vi "多道分析仪.vi"() -> ()   [LabVIEW 2014]
uses:
  <vilib>/Utility/miscctls.llb/LVPointDoubleTypeDef.ctl
  <vilib>/Utility/file.llb/Read From Spreadsheet File (DBL).vi
  <vilib>/Utility/file.llb/Write To Spreadsheet File (DBL).vi
  <vilib>/Analysis/NI_AAL_SigProc.lvlib
  <vilib>/Analysis/NI_AALPro.lvlib
panel:
  out "状态：本次测量和上次未完成测量时间和":dbl
  out "状态：本次测试已测时间":dbl
  out "状态：上次未完成测试的已测时间":dbl
  out "变量：每次测量计划用时":u16=3600
  out "设置：幅度谱总道数 2":u32=4096
  out "变量：实时计数":i32
  out "变量：剩余使用时间":dbl
  out "center":dbl caption="中心"
  in  "设置：信号极性（正T）":bool=TRUE
  in  "数据缓存索引":u32
  out "变量 : 实时总计数":u64
  out "设置 ： 修正文件路径":path
  out "变量 ： 上次测量总计数":u32
  out "变量：上次测量原始数据":dbl[](array[numeric])
  out "状态：已测时间":dbl
  out "状态：测量开始时间":u32
  out "状态：刷新次数":i32
  in  "状态：停止变量":bool=TRUE
  out "变量：上次测量时间":dbl
  out "变量：原始数据":dbl[](array[numeric])
  out "MCA道宽修正数组":ext[](array[numeric])
  in  "设置：寻峰灵敏度":i32=3 caption="宽度" min=3
  in  "设置：甄别前阈值":u16=10000
  in  "设置：甄别后阈值":u16=9000
  in  "设置：刷新频率":u16
  in  "设置：测量时间":u16
  out "结果：净面积":dbl=1313865.0
  out "结果：半高宽":dbl=218.0
  out "结果：峰位":dbl=1585.0 caption="中心"
  in  "按钮_游标":bool caption="游标"
  in  "按钮_寻峰":T1 caption="寻峰"
  in  "按钮_右移":bool caption="右移"
  in  "按钮_还原":bool caption="还原"
  in  "按钮_放大":bool caption="放大"
  in  "按钮_左移":bool caption="左移"
  out "变量：感兴区终点道址":dbl=-1.0
  in  "显示：列表显示内容":string[](array[string])=["", "0秒", "正", "9000", "10000", "", "", "2014年3月7日", "0:56:44", "0秒", "0", "", "", "", "", "", "", "", "", "", "", ""]
  out "变量：感兴区起点道址":dbl=-1.0
  out "设置：幅度谱总道数":u32=4096
  in  "变量：图像缓存数组":dbl[][](array[numeric])
  in  "按钮_退出":bool caption="退出"
  in  "按钮_帮助":bool caption="帮助"
  in  "按钮_复位":bool caption="复位"
  in  "按钮_停止":bool caption="停止"
  in  "按钮_开始":bool caption="开始"
  in  "按钮_设置":bool caption="设置"
  in  "按钮_保存":bool caption="保存"
  in  "按钮_打开":bool caption="打开"
  out "显示：波形图":dbl[][](graph)
  out "显示：列表框":T2=6
  out "显示：波形图_预览":dbl[][](graph)
  out "状态栏_仪器状态":T3="核电子学硬件平台未连接" caption="状态栏"
  out "状态栏_剩余使用时间":T3="0" caption="剩余使用时间："
  out "状态栏_计数率":T3="0" caption="实时计数率："
  out "状态栏_游标状态":T3="隐藏" caption="游标状态："
  out "状态栏_游标计数":T3="0" caption="游标计数："
  out "状态栏_游标道址":T3="0" caption="游标道址："
  out "状态栏_测量状态":T3="停止" caption="测量状态："
  out "状态栏_日期":T3="2014/3/7   0:56:56" caption="日期"
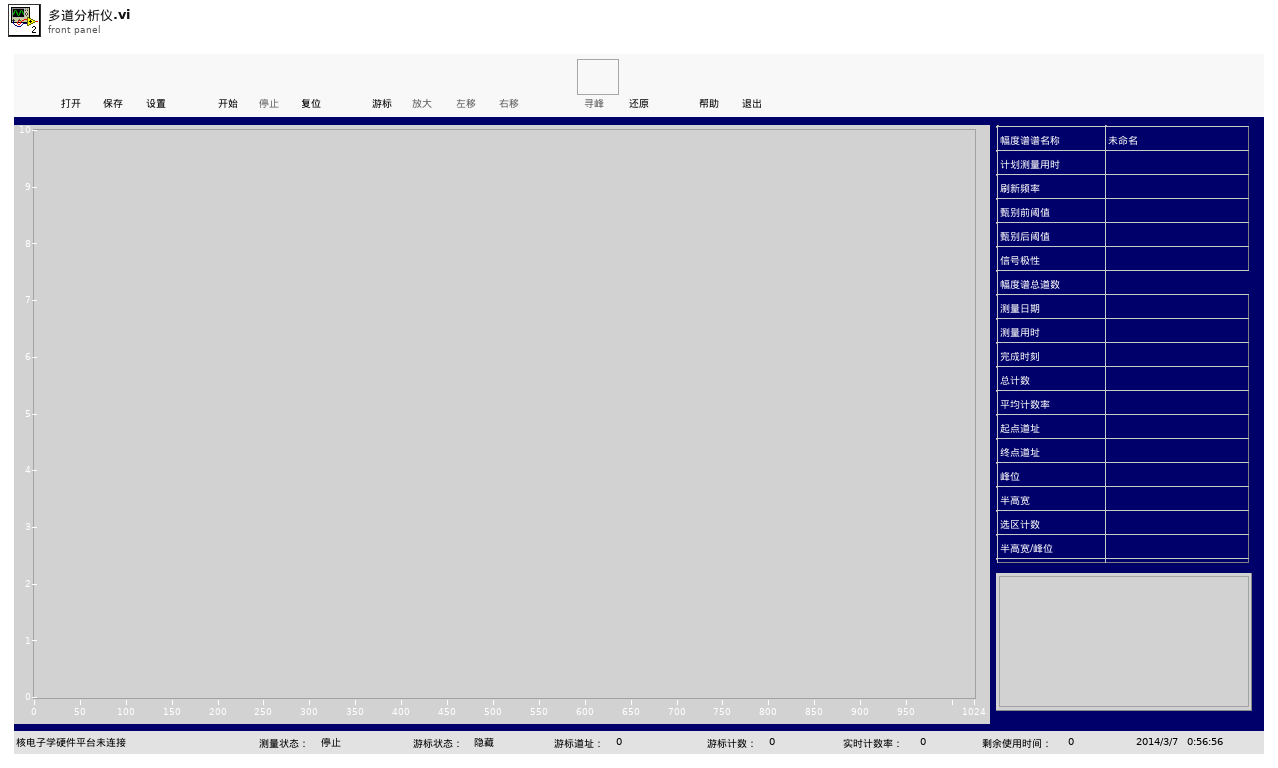
[diagram p1: front panel]
types:
  T1 = typedef "寻峰控件.ctl" = bool
  T2 = typedef "透明表格.ctl" = i32
  T3 = typedef "透明字符串.ctl" = string
  T4 = typedef "枚举常量_状态机.ctl" = enum16{"初始化", "等待", "完成"}
  T5 = typedef "LVPointDoubleTypeDef.ctl" = cluster{"X":dbl, "Y":dbl}
  T6 = enum8{"Enabled", "Disabled", "Disabled and Grayed Out"}
  T7 = enum16{"open", "open or create", "create or replace", "create", "open (read-only)"}
  T8 = typedef "eventvkey.ctl" = enum16{"ASCII", "Enter", "Return", "Shift", "Ctrl", "Alt", "Cmd", "Opt", "Caps", "NumLock", "Clear", "Break", "Up", "Down", "Left", "Right", "Insert", "Delete", "Home", "End", "PageUp", "PageDown", "Escape", "Help", "Pause", "ScrollLock", "F1", "F2", "F3", "F4", "F5", "F6", "F7", "F8", "F9", "F10", "F11", "F12", "F13", "F14", "F15", "F16", "F17", "F18", "F19", "F20", "F21", "F22", "F23", "F24", "Play", "VolumeUp", "VolumeDown", "Mute", "Two Byte Char"}
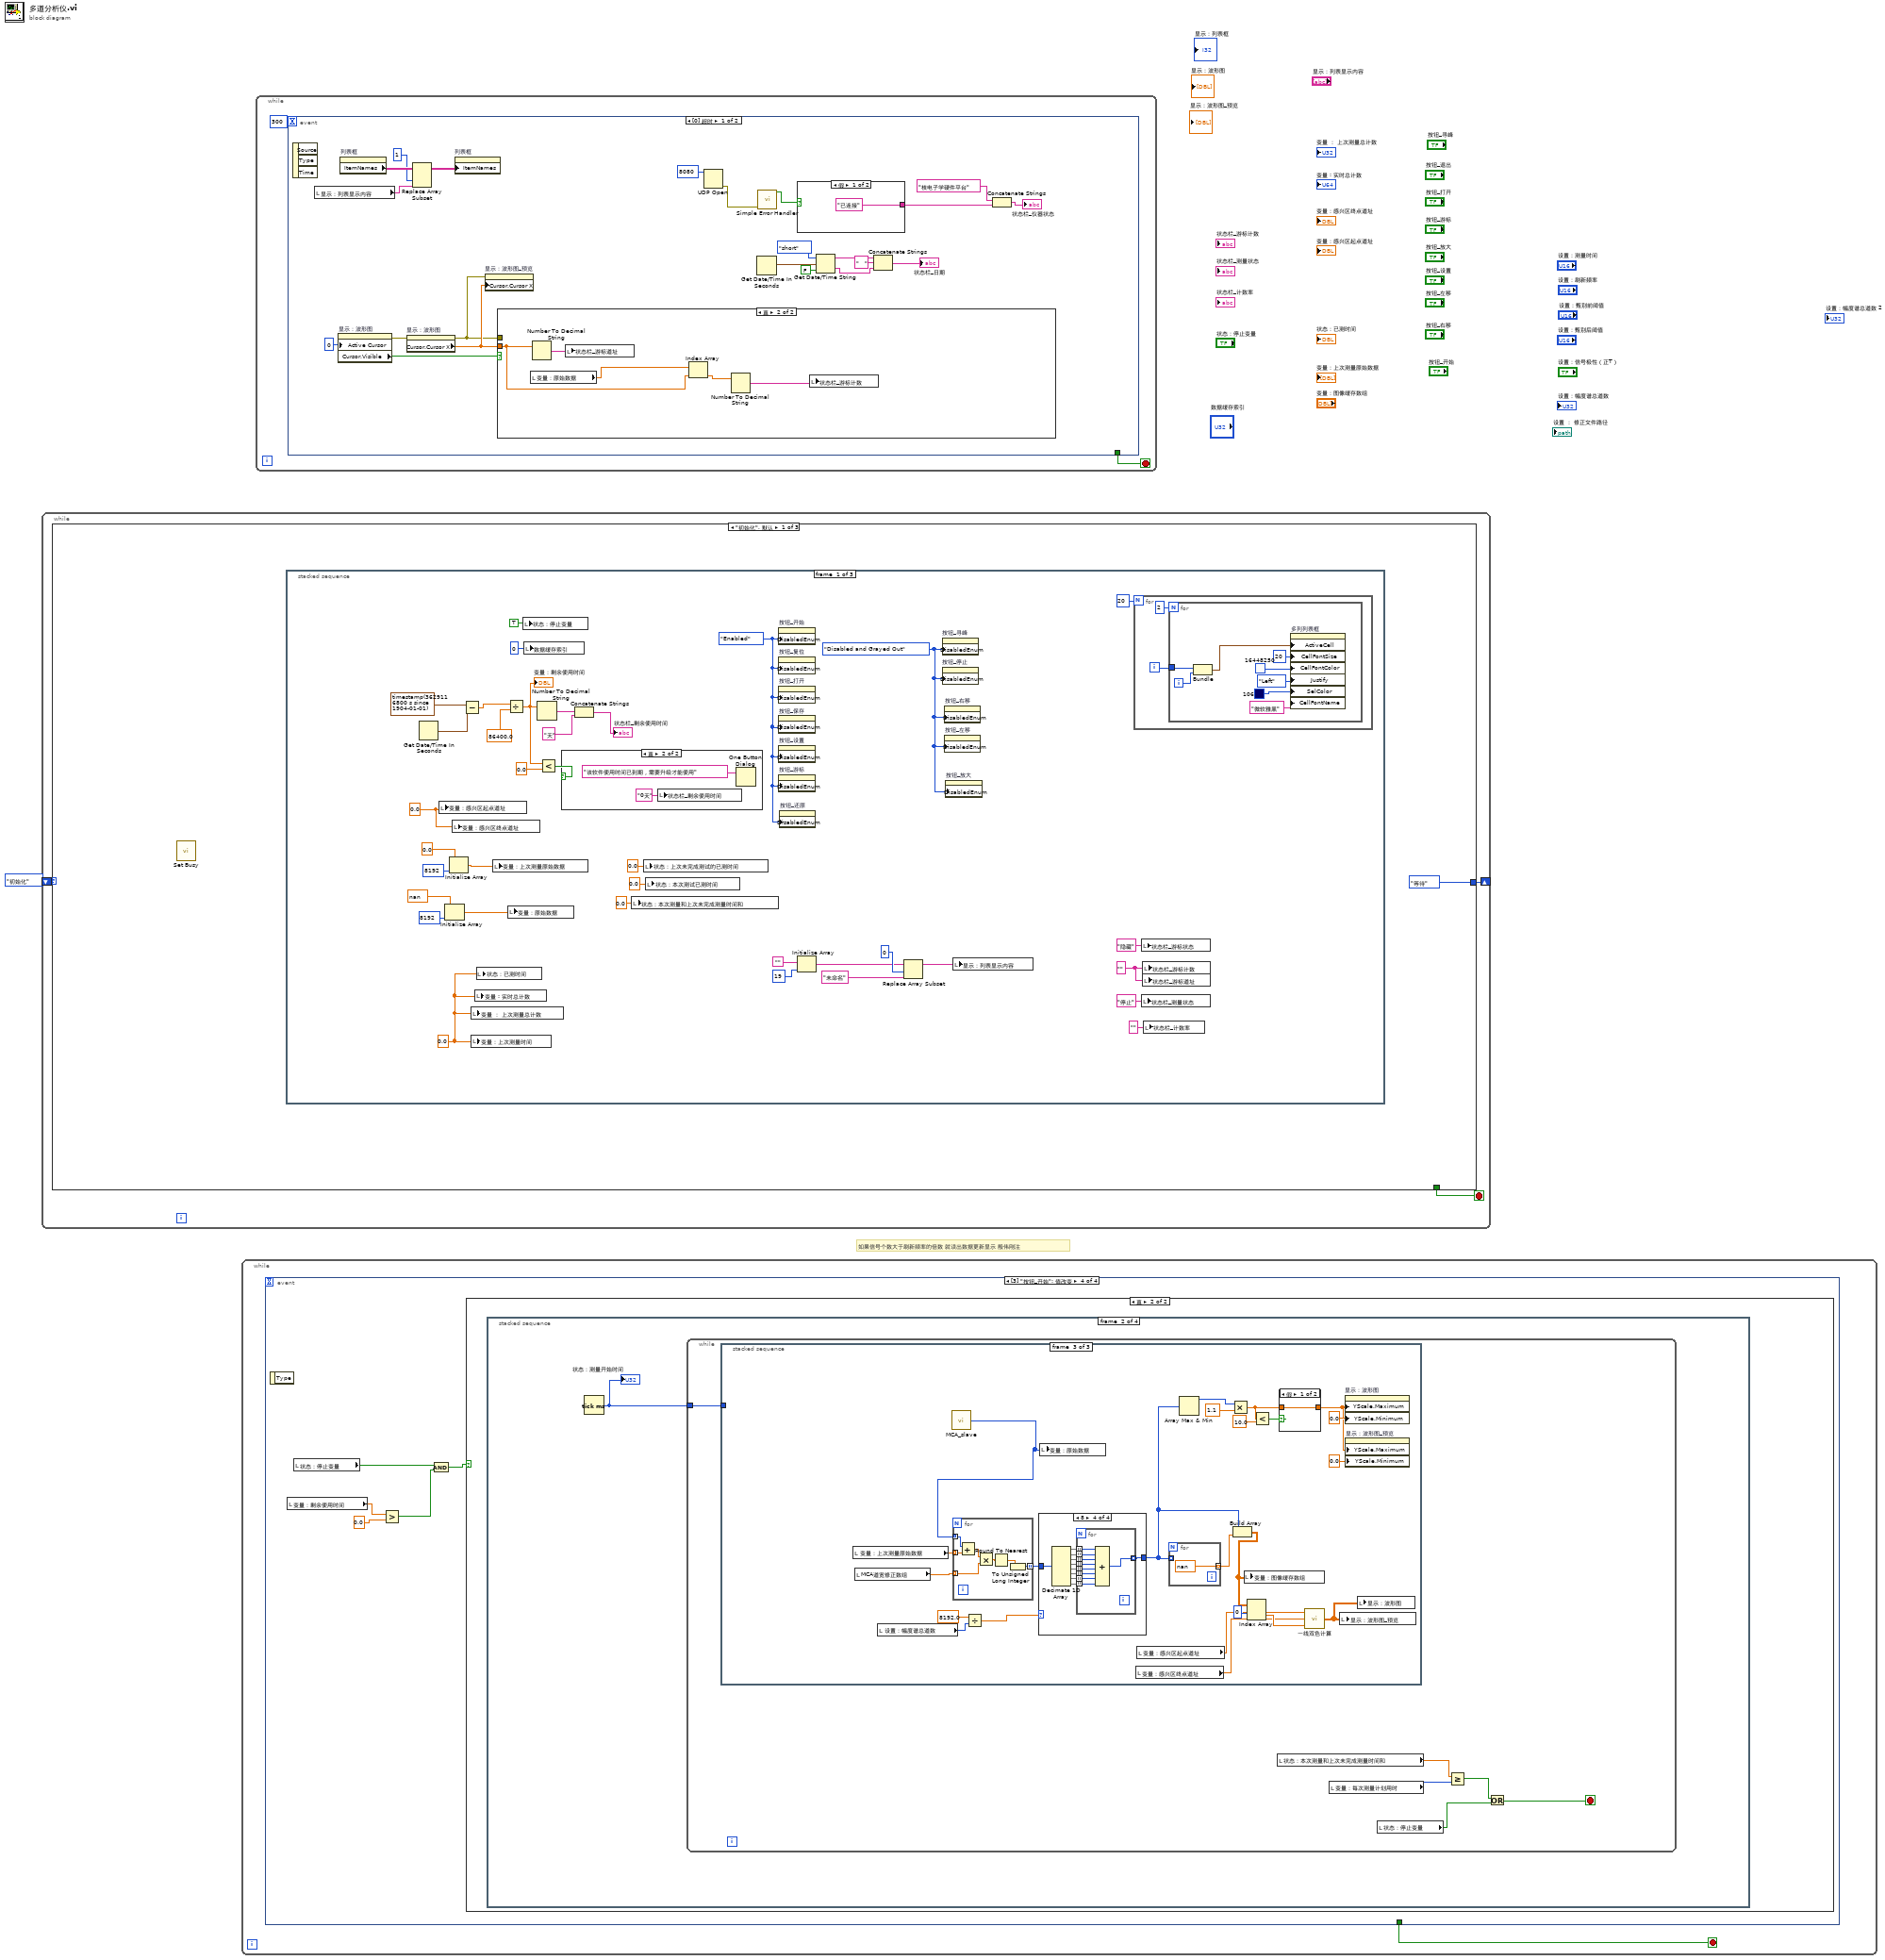
[diagram p0: block diagram]
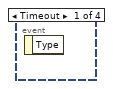
[diagram p2: hidden frame]
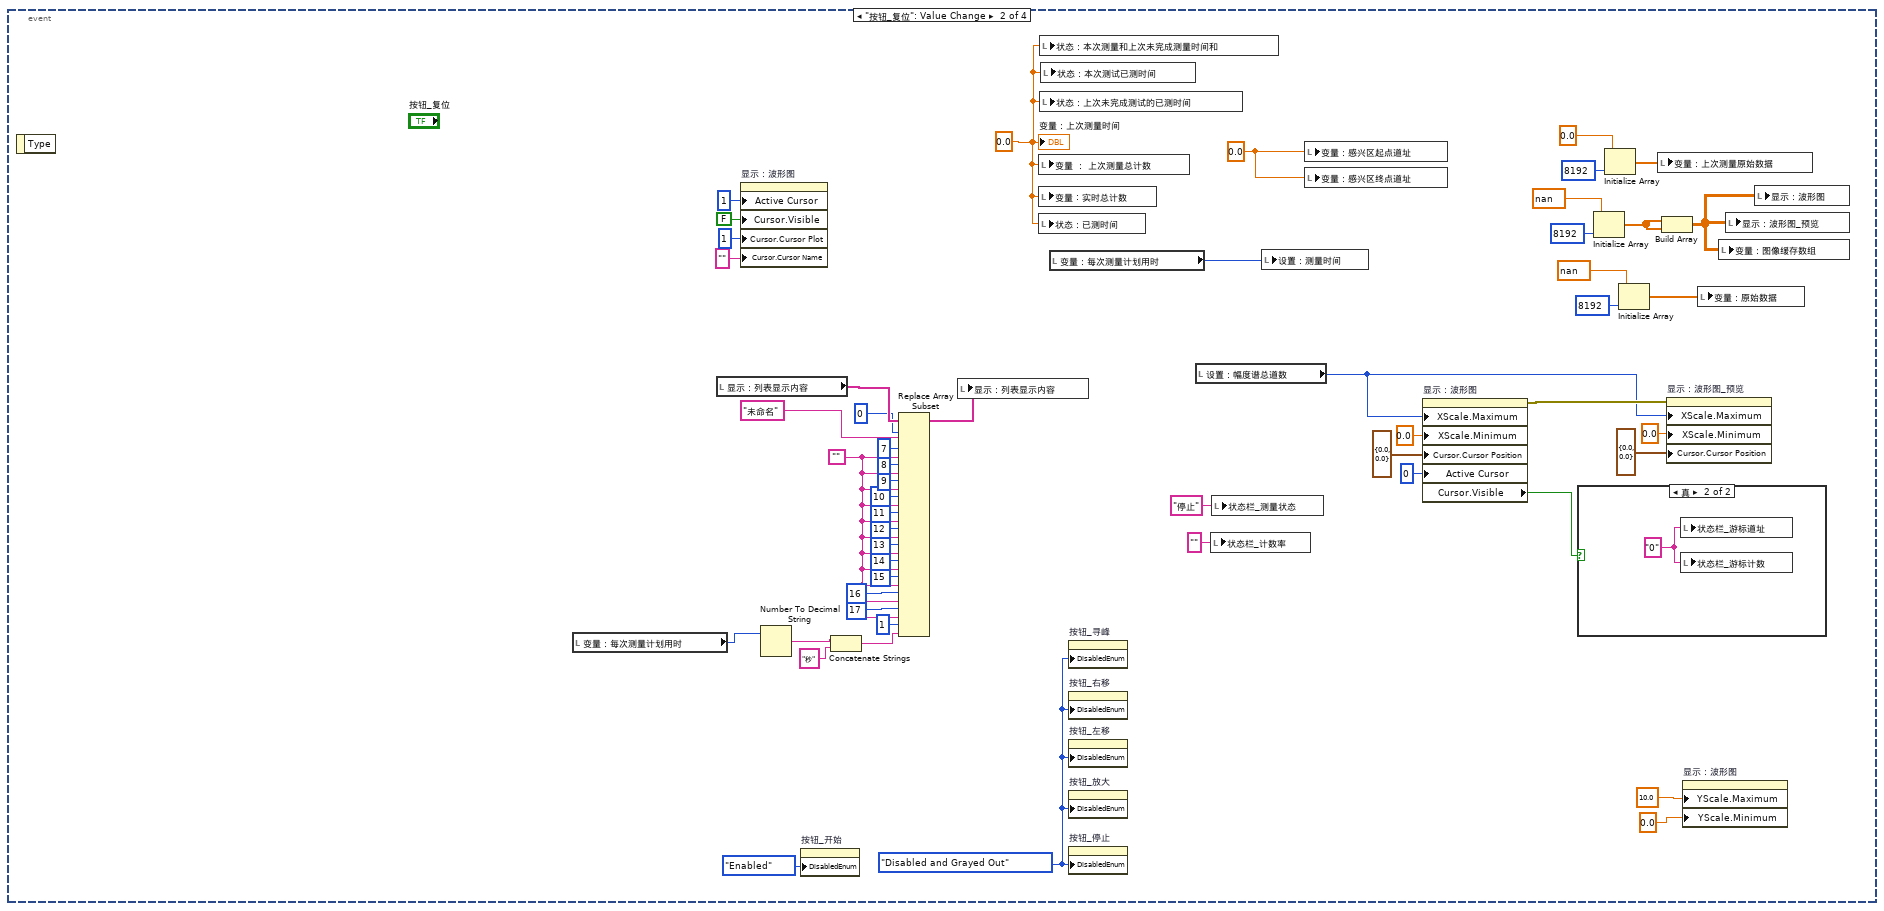
[diagram p3: hidden frame]
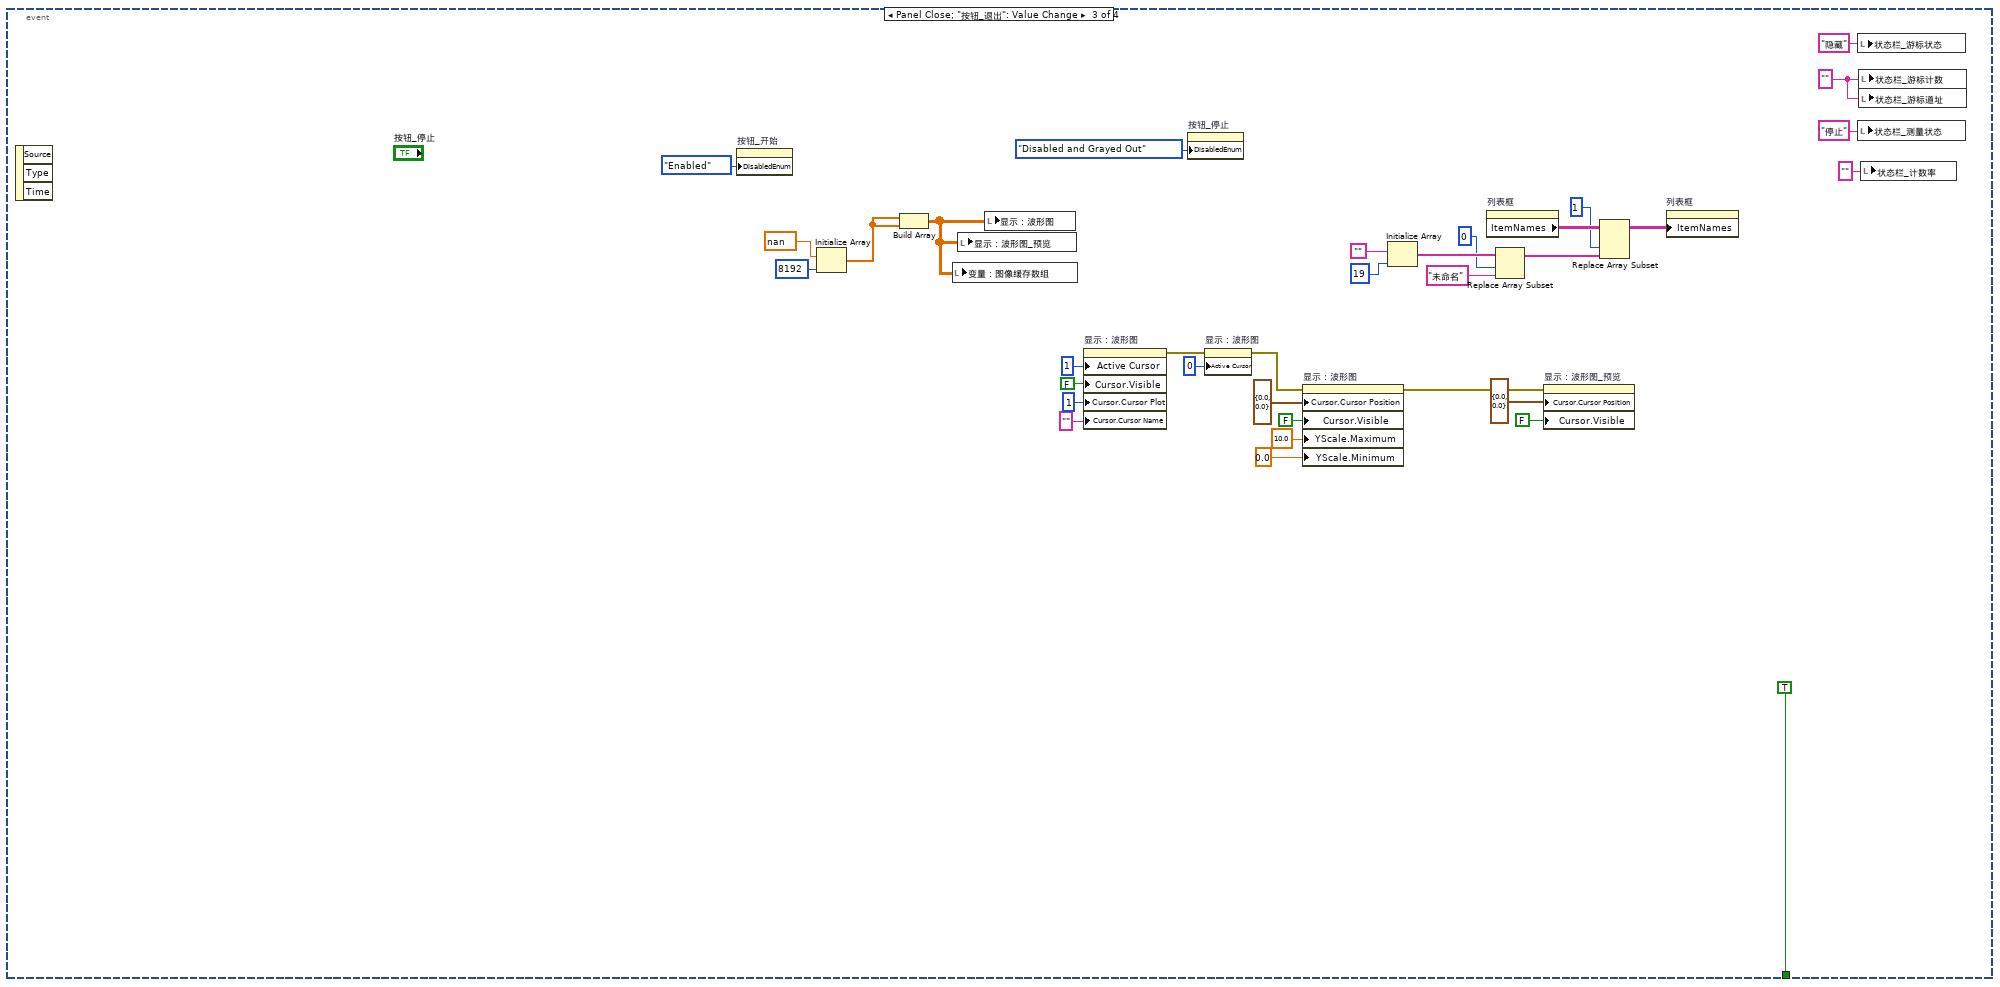
[diagram p5: hidden frame]
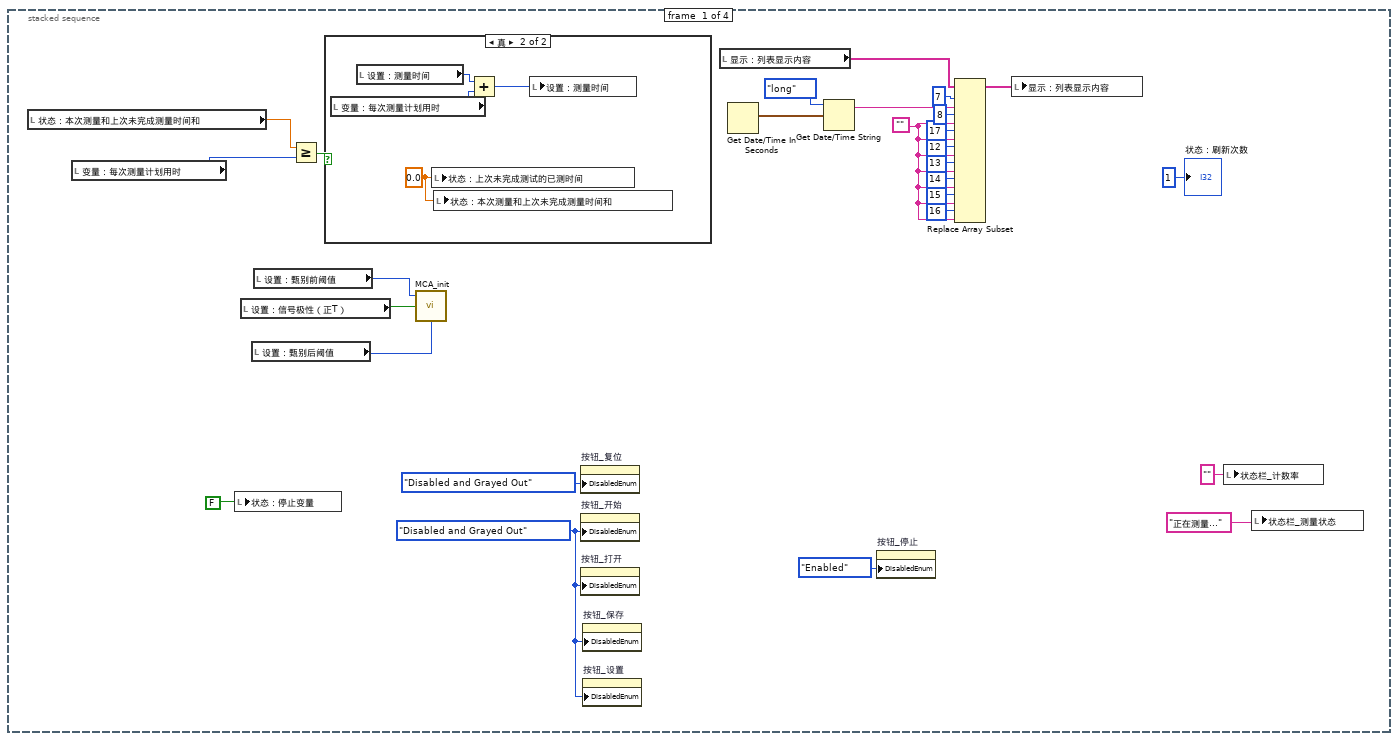
[diagram p7: hidden frame]
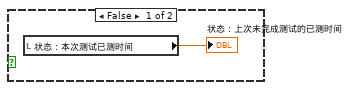
[diagram p8: hidden frame]
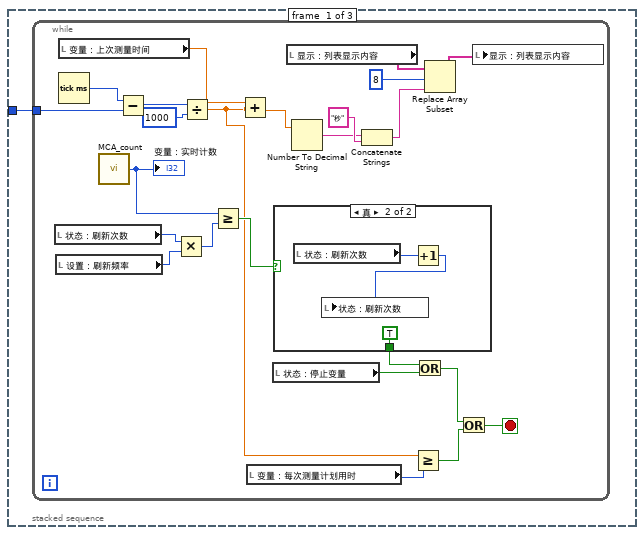
[diagram p9: hidden frame]
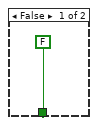
[diagram p10: hidden frame]
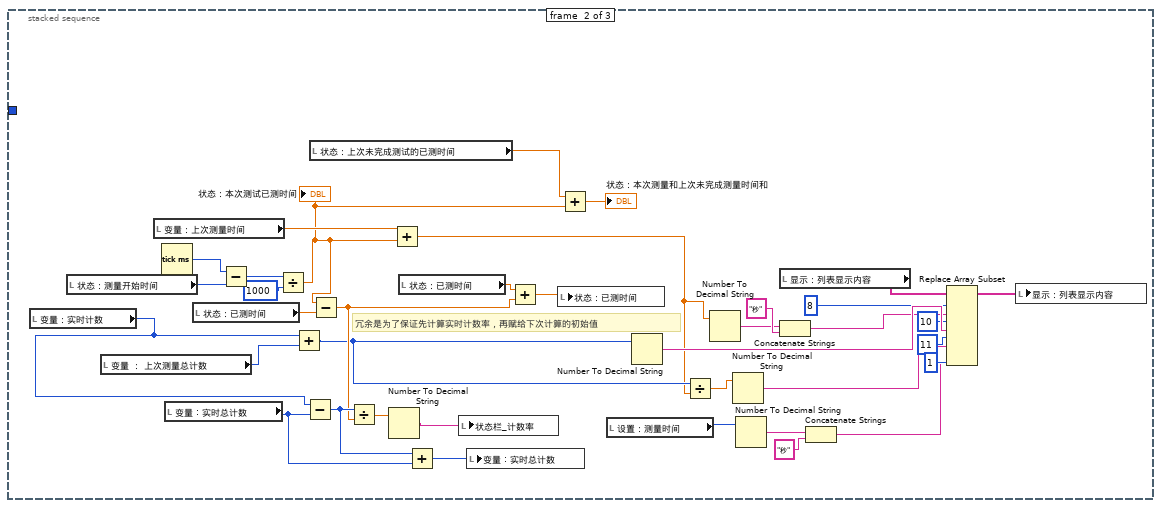
[diagram p11: hidden frame]
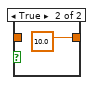
[diagram p12: hidden frame]
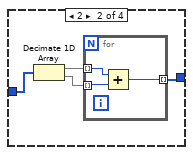
[diagram p14: hidden frame]
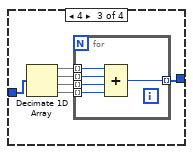
[diagram p15: hidden frame]
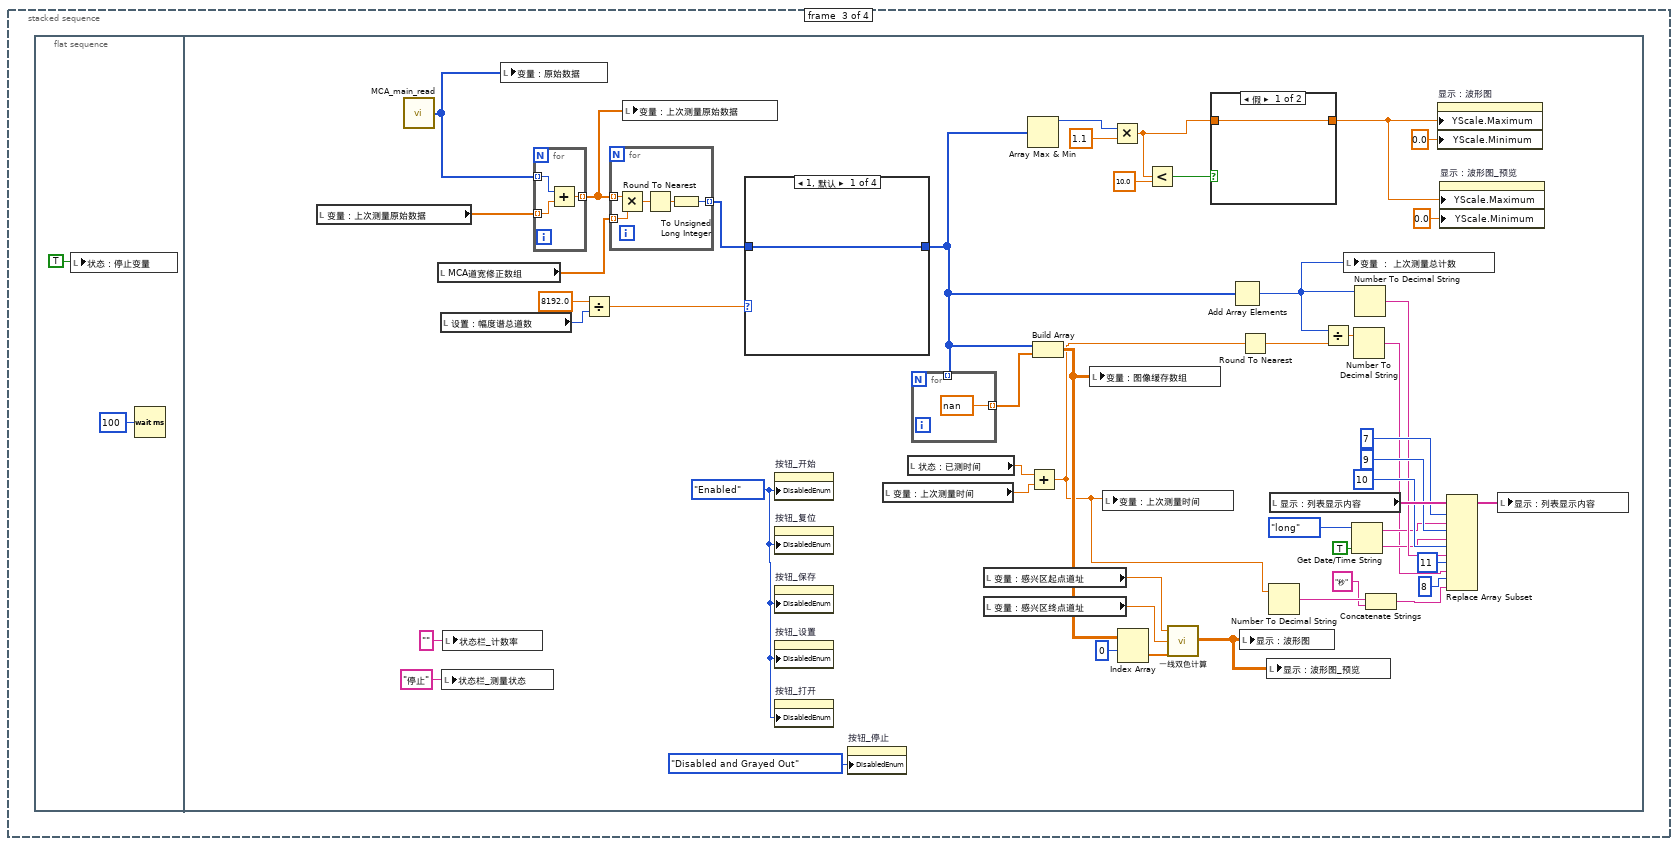
[diagram p16: hidden frame]
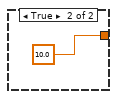
[diagram p17: hidden frame]
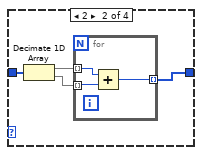
[diagram p18: hidden frame]
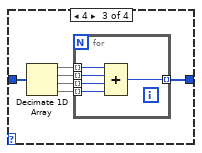
[diagram p19: hidden frame]
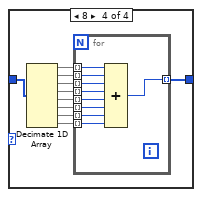
[diagram p20: hidden frame]
diagram:
  # "如果信号个数大于刷新频率的倍数 就读出数据更新显示 殷伟刚注"
  n1 = while {
    shift-right: [w3] -> _
    shift-left: 枚举常量_状态机."初始化" ("枚举") -> [w4]
    stop <- w2 stop-if-true
    n2 = case shown="\"初始化\", 默认" w4 {
      tunnel: [枚举常量_状态机."等待" ("枚举") w121 枚举常量_状态机."完成" ("枚举")] -> w3
      tunnel: [_ _ TRUE] -> w2
      frame "初始化", Default {
        n3 = call <vilib>:"Set Busy.vi"() -> ()  [unwired: 10 in, 2 out]
        n4 = stacked-sequence {
          frame #0 {
            w28 = 0.0
            w25 = 0.0 ("变量：已测量时间")
            w30 = T6."Enabled" ("禁用")
            w38 = T3 "" ("状态栏_游标计数")
            w20 = T6."Disabled and Grayed Out" ("禁用")
            n5 = Get Date/Time In Seconds() -> (seconds since 1Jan1904=w12:timestamp)
            n6 = local write "变量：感兴区起点道址"(w28) -> ()
            n7 = Initialize Array(nan ("元素"), 8192 ("维数大小")) -> (w21:dbl[])
            n8 = Initialize Array(0.0 ("元素"), 8192 ("维数大小")) -> (w24:dbl[])
            n9 = local write "变量：感兴区终点道址"(w28) -> ()
            n10 = Subtract(x=timestamp(3629116800 s since 1904-01-01), y=w12) -> (x-y=w14:dbl)
            n11 = local write "变量 ： 上次测量总计数"(w25) -> ()
            n12 = local write "变量：上次测量时间"(w25) -> ()
            n13 = local write "变量 : 实时总计数"(w25) -> ()
            n14 = local write "状态：已测时间"(w25) -> ()
            n15 = local write "变量：上次测量原始数据"(w24) -> ()
            n16 = Divide(x=w14, y=86400.0) -> (x/y=w11:dbl)
            "变量：剩余使用时间" <- w11
            n17 = local write "变量：原始数据"(w21) -> ()
            n18 = local write "状态：停止变量"(TRUE ("停止变量")) -> ()
            n19 = local write "数据缓存索引"(u32 0 ("数据缓存索引")) -> ()
            n20 = Number To Decimal String(number=w11) -> (decimal integer string=w16:string)  [unwired: 1 in]
            n21 = Less?(x=w11, y=0.0) -> (x < y?=w9:bool)
            n22 = case shown="真" w9 {
              frame False {
              }
              frame True {
                n23 = local write "状态栏_剩余使用时间"(T3 "0天" ("状态栏_剩余使用时间")) -> ()
                n24 = One Button Dialog(message="该软件使用时间已到期，需要升级才能使用" ("消息")) -> ()  [unwired: 1 in, 1 out]
              }
            }
            n25 = Concatenate Strings(w16, "天" ("字符串")) -> (→"状态栏_剩余使用时间":string)
            n26 = local write "状态：本次测量和上次未完成测量时间和"(0.0 ("状态：本次测量和上次未完成测量时间和")) -> ()
            n27 = local write "状态：上次未完成测试的已测时间"(0.0 ("状态：上次未完成测试的已测时间")) -> ()
            n28 = local write "状态：本次测试已测时间"(0.0 ("状态：本次测试已测时间")) -> ()
            n29 = property on="按钮_开始" class="Bool"("DisabledEnum"=w30) -> ()  [unwired: 2 in, 2 out]
            n30 = property on="按钮_复位" class="Bool"("DisabledEnum"=w30) -> ()  [unwired: 2 in, 2 out]
            n31 = property on="按钮_打开" class="Bool"("DisabledEnum"=w30) -> ()  [unwired: 2 in, 2 out]
            n32 = property on="按钮_保存" class="Bool"("DisabledEnum"=w30) -> ()  [unwired: 2 in, 2 out]
            n33 = property on="按钮_设置" class="Bool"("DisabledEnum"=w30) -> ()  [unwired: 2 in, 2 out]
            n34 = property on="按钮_游标" class="Bool"("DisabledEnum"=w30) -> ()  [unwired: 2 in, 2 out]
            n35 = property on="按钮_还原" class="Bool"("DisabledEnum"=w30) -> ()  [unwired: 2 in, 2 out]
            n36 = Initialize Array("", 19 ("维数大小")) -> (w31:string[])
            n37 = Replace Array Subset(array=w31, new element="未命名" ("新元素/子数组"), index=0 ("索引")) -> (w36:string[])
            n38 = property on="按钮_寻峰" class="Bool"("DisabledEnum"=w20) -> ()  [unwired: 2 in, 2 out]
            n39 = property on="按钮_停止" class="Bool (严格)"("DisabledEnum"=w20) -> ()  [unwired: 2 in, 2 out]
            n40 = property on="按钮_右移" class="Bool"("DisabledEnum"=w20) -> ()  [unwired: 2 in, 2 out]
            n41 = property on="按钮_左移" class="Bool"("DisabledEnum"=w20) -> ()  [unwired: 2 in, 2 out]
            n42 = property on="按钮_放大" class="Bool"("DisabledEnum"=w20) -> ()  [unwired: 2 in, 2 out]
            n43 = local write "显示：列表显示内容"(w36) -> ()
            n44 = for {
              N: 20 -> [_]
              i -> [w44]
              n45 = for {
                N: 2 -> [_]
                tunnel: w44 -> [w52]
                i -> [w53]
                n46 = Bundle(w52, w53) -> (w51:cluster{i32, i32})  [unwired: 1 in]
                n47 = property on="多列列表框" class="MCListbox (严格)"("ActiveCell"=w51, "CellFontSize"=u32 20 ("活动单元格:单元格字体:字号"), "CellFontColor"=u32 16448250 ("Color"), "Justify"=enum16{"Left", "Center", "Right"}."Left" ("活动单元格:单元格对齐"), "SelColor"=u32 106 ("Color"), "CellFontName"="微软雅黑" ("活动单元格:单元格字体:名称")) -> ()  [unwired: 2 in, 2 out]
              }
            }
            n48 = local write "状态栏_游标状态"(T3 "隐藏" ("状态栏_游标状态")) -> ()
            n49 = local write "状态栏_测量状态"(T3 "停止" ("状态栏_测量状态")) -> ()
            n50 = local write "状态栏_游标计数"(w38) -> ()
            n51 = local write "状态栏_游标道址"(w38) -> ()
            n52 = local write "状态栏_计数率"(T3 "" ("状态栏_计数率")) -> ()
          }
          frame #1 {
            # "此处得到MCA道宽不均匀修正数组"
            n53 = call "MCA_ReadConfig.vi"() -> ("数据刷新频率"=w57:u16, "测量最多花费的时间（秒）："=w58:u16, "甄别后阈值"=w59:u16, "甄别前阈值"=w60:u16, "寻峰灵敏度"=w56:u16, "最大道数"=w54:u16, "数据文件路径"=w55:path, "信号极性"=w61:bool)  [unwired: 3 in, 1 out]
            "变量：每次测量计划用时" <- w58
            n54 = local write "设置：信号极性（正T）"(w61) -> ()
            n55 = local write "设置：幅度谱总道数"(w54) -> ()
            n56 = local write "设置：甄别前阈值"(w60) -> ()
            n57 = local write "设置：甄别后阈值"(w59) -> ()
            n58 = local write "设置：测量时间"(w58) -> ()
            n59 = local write "设置：刷新频率"(w57) -> ()
            n60 = local write "设置：寻峰灵敏度"(w56) -> ()
            n61 = Equal?(x=w55, y=path "") -> (x = y?=w83:bool)
            n62 = case shown="真" w83 {
              tunnel: w55 -> [w88 _]
              tunnel: [w86 w89] -> w62
              frame False {
                n63 = call-poly <vilib>:"Read From Spreadsheet File.vi"("transpose (no:F)"=TRUE, "file path (dialog if empty)"=w88) -> ("first row"=w86:dbl[])  [unwired: 5 in, 4 out]
              }
              frame True {
                n64 = Initialize Array(1.0 ("元素"), 8192 ("维数大小")) -> (w89:dbl[])
              }
            }
            "MCA道宽修正数组" <- w62
            n65 = local write "设置 ： 修正文件路径"(w55) -> ()
            n66 = property on="显示：波形图" class="WFGraph (严格)"("Active Cursor"=u32 1 ("活动游标"), "Cursor.Visible"=FALSE ("游标.可见"), "Cursor.Cursor Plot"=1 ("游标.游标关联曲线"), "Cursor.Cursor Name"="" ("游标.游标名")) -> (error out=w66:errorcluster)  [unwired: 2 in, 1 out]
            n67 = property on="显示：波形图" class="WFGraph (严格)"(error in=w66, "Active Cursor"=u32 0 ("活动游标")) -> (error out=w71:errorcluster)  [unwired: 1 in, 1 out]
            n68 = property on="显示：波形图" class="WFGraph (严格)"(error in=w71, "XScale.Maximum"=w54, "XScale.Minimum"=0.0 ("X标尺.范围:最小值"), "Cursor.Cursor Position"=T5 {"X"=0.0, "Y"=0.0} ("游标.游标位置"), "Cursor.Visible"=FALSE ("游标.可见"), "YScale.Maximum"=10.0 ("Y标尺.范围:最大值"), "YScale.Minimum"=0.0 ("Y标尺.范围:最小值")) -> (error out=w74:errorcluster)  [unwired: 1 in, 1 out]
            n69 = Initialize Array(nan ("元素"), w54) -> (w82:dbl[])
            n70 = for {
              tunnel: w82 -> [_] mode=indexing
              tunnel: [nan] -> w79 mode=indexing
            }
            n71 = property on="显示：波形图_预览" class="WFGraph (严格)"(error in=w74, "XScale.Maximum"=w54, "XScale.Minimum"=0.0 ("X标尺.范围:最小值"), "Cursor.Cursor Position"=T5 {"X"=0.0, "Y"=0.0} ("游标.游标位置"), "Cursor.Visible"=FALSE ("游标.可见")) -> ()  [unwired: 1 in, 2 out]
            n72 = Build Array(w82, w79) -> (w80:dbl[][])
            n73 = local write "显示：波形图_预览"(w80) -> ()
            n74 = local write "变量：图像缓存数组"(w80) -> ()
            n75 = local write "显示：波形图"(w80) -> ()
          }
          frame #2 {
            n76 = local read "设置：信号极性（正T）"() -> (w99:bool)
            n77 = local read "设置：寻峰灵敏度"() -> (w102:i32)
            n78 = local read "设置：幅度谱总道数"() -> (w94:u32)
            n79 = local read "设置：测量时间"() -> (w106:u16)
            n80 = local read "设置：刷新频率"() -> (w105:u16)
            n81 = local read "设置：甄别后阈值"() -> (w103:u16)
            n82 = local read "设置：甄别前阈值"() -> (w104:u16)
            n83 = case shown="假" w99 {
              tunnel: ["负" ("字符串") "正" ("字符串")] -> w98
              frame False {
              }
              frame True {
              }
            }
            n84 = Number To Decimal String(number=w102) -> (decimal integer string=w96:string)  [unwired: 1 in]
            n85 = Number To Decimal String(number=w94) -> (decimal integer string=w93:string)  [unwired: 1 in]
            n86 = Number To Decimal String(number=w106) -> (decimal integer string=w111:string)  [unwired: 1 in]
            n87 = Number To Decimal String(number=w103) -> (decimal integer string=w100:string)  [unwired: 1 in]
            n88 = Number To Decimal String(number=w105) -> (decimal integer string=w116:string)  [unwired: 1 in]
            n89 = Number To Decimal String(number=w104) -> (decimal integer string=w101:string)  [unwired: 1 in]
            n90 = Concatenate Strings(w111, "秒" ("字符串")) -> (w112:string)
            n91 = Concatenate Strings(w116, "个/次" ("字符串")) -> (w118:string)
            n92 = local read "显示：列表显示内容"() -> (w108:string[])
            n93 = Replace Array Subset(array=w108, new element #1=w112, index #1=1 ("索引"), new element #2=w118, index #2=2 ("索引"), new element #3=w101, index #3=3 ("索引"), new element #4=w100, index #4=4 ("索引"), new element #5=w98, index #5=5 ("索引"), new element #6=w93, index #6=6 ("索引"), new element #7=w96, index #7=18 ("索引")) -> (w109:string[])
            n94 = local write "显示：列表显示内容"(w109) -> ()
          }
        }
      }
      frame "等待" {
        n95 = call <vilib>:"Unset Busy.vi"() -> ()  [unwired: 11 in, 1 out]
        n96 = event shown="[5] \"按钮_打开\": 值改变" {
          selector: _ -> [_ _ _ _ _ _ _ _ _ _ _ _ _ _ _ _ _]
          dyn-events: _ -> [_ _ _ _ _ _ _ _ _ _ _ _ _ _ _ _ _]
          timeout: _ -> [_ _ _ _ _ _ _ _ _ _ _ _ _ _ _ _ _]
          tunnel: [枚举常量_状态机."等待" ("枚举") 枚举常量_状态机."等待" ("枚举") 枚举常量_状态机."完成" ("枚举") 枚举常量_状态机."等待" ("枚举") 枚举常量_状态机."等待" ("枚举") 枚举常量_状态机."等待" ("枚举") 枚举常量_状态机."等待" ("枚举") 枚举常量_状态机."等待" ("枚举") 枚举常量_状态机."等待" ("枚举") 枚举常量_状态机."等待" ("枚举") 枚举常量_状态机."等待" ("枚举") 枚举常量_状态机."等待" ("枚举") 枚举常量_状态机."等待" ("枚举") 枚举常量_状态机."等待" ("枚举") 枚举常量_状态机."等待" ("枚举") 枚举常量_状态机."等待" ("枚举") 枚举常量_状态机."等待" ("枚举")] -> w121
          event Timeout {
            n97 = event-data() -> ()  [unwired: 1 in, 3 out]
          }
          event "按钮_帮助": Value Change {
            n98 = event-data() -> ()  [unwired: 1 in, 6 out]
            n99 = call "显示对话框信息"() -> ("软件介绍"=w123:bool)  [unwired: 10 in, 1 out]
            n100 = case shown="真" w123 {
              frame False {
              }
              frame True {
                n101 = call "显示对话框信息2"() -> ()  [unwired: 10 in, 2 out]
              }
            }
          }
          event "按钮_退出": Value Change {
            n102 = event-data() -> ()  [unwired: 1 in, 6 out]
            n103 = local write "状态：停止变量"(TRUE ("停止变量")) -> ()
          }
          event "按钮_停止": Value Change {
            w130 = T6."Enabled" ("禁用")
            n104 = event-data() -> ()  [unwired: 1 in, 6 out]
            n105 = property on="按钮_复位" class="Bool"("DisabledEnum"=w130) -> ()  [unwired: 2 in, 2 out]
            n106 = property on="按钮_开始" class="Bool"("DisabledEnum"=T6."Enabled" ("禁用")) -> ()  [unwired: 2 in, 2 out]
            n107 = property on="按钮_打开" class="Bool"("DisabledEnum"=w130) -> ()  [unwired: 2 in, 2 out]
            n108 = property on="按钮_保存" class="Bool"("DisabledEnum"=w130) -> ()  [unwired: 2 in, 2 out]
            n109 = property on="按钮_设置" class="Bool"("DisabledEnum"=w130) -> ()  [unwired: 2 in, 2 out]
            n110 = local write "状态：停止变量"(TRUE ("停止变量")) -> ()
            n111 = property on="按钮_停止" class="Bool (严格)"("Value"=FALSE ("停止"), "DisabledEnum"=T6."Disabled and Grayed Out" ("禁用")) -> ()  [unwired: 2 in, 2 out]
          }
          event "显示：波形图": Cursor Move {
            n112 = event-data() -> ()  [unwired: 1 in, 9 out]
            n113 = property on="显示：波形图" class="WFGraph (严格)"() -> ("Cursor.Cursor Position"=w140:T5)  [unwired: 2 in, 2 out]
            n114 = property on="显示：波形图_预览" class="WFGraph (严格)"("Cursor.Cursor Position"=w140) -> ()  [unwired: 2 in, 2 out]
            n115 = Unbundle By Name(w140) -> ("Cursor X"=w137:dbl, "Cursor Y"=w136:dbl)
            n116 = Number To Decimal String(number=w137) -> (decimal integer string=→"状态栏_游标道址":string)  [unwired: 1 in]
            n117 = Number To Decimal String(number=w136) -> (decimal integer string=w135:string)  [unwired: 1 in]
            n118 = Equal?(x=w135, y="NaN") -> (x = y?=w141:bool)
            n119 = case shown="真" w141 {
              tunnel: [w143 w149] -> w138
              tunnel: w136 -> [w143 _]
              frame False {
              }
              frame True {
                n120 = property on="显示：波形图" class="WFGraph (严格)"() -> (error out=w150:errorcluster, "Cursor.Cursor Plot"=w146:i32)  [unwired: 2 in, 1 out]
                n121 = Equal To 0?(x=w146) -> (x = 0?=w147:bool)
                n122 = Select(t=1.0, s=w147, f=0.0) -> (s? t:f=w148:dbl)
                n123 = property on="显示：波形图" class="WFGraph (严格)"(error in=w150, "Cursor.Cursor Plot"=w148) -> ("Cursor.Cursor Y"=w149:dbl)  [unwired: 1 in, 2 out]
              }
            }
            n124 = Number To Decimal String(number=w138) -> (decimal integer string=w133:string)  [unwired: 1 in]
            n125 = local write "状态栏_游标计数"(w133) -> ()
          }
          event "按钮_打开": Value Change {
            n126 = event-data() -> ()  [unwired: 1 in, 1 out]
            n127 = call "MCA_OpenDialog.vi"() -> ("要打开的数据文件路径： 2"=w151:path, "是否取消？"=w152:bool)  [unwired: 10 in]
            n128 = case shown="假" w152 {
              tunnel: w151 -> [w154 _]
              frame False {
                n129 = Strip Path(path=w154) -> (name=w161:string)  [unwired: 1 out]
                n130 = String Length(string=w161) -> (length=w160:i32)
                n131 = Subtract(x=w160, y=4) -> (x-y=w158:i32)
                n132 = String Subset(string=w161, offset (0)=w158, length (rest)=w160) -> (substring=w157:string)
                n133 = Equal?(x=w157, y="tdms") -> (x = y?=w155:bool)
                n134 = case shown="真" w155 {
                  tunnel: w154 -> [w163 w195]
                  frame False {
                    n135 = Strip Path(path=w163) -> (name=w162:string)  [unwired: 1 out]
                    n136 = String Length(string=w162) -> (length=w169:i32)
                    n137 = Subtract(x=w169, y=4) -> (x-y=w167:i32)
                    n138 = String Subset(string=w162, offset (0)=w167, length (rest)=w169) -> (substring=w166:string)
                    n139 = Equal?(x=w166, y=".txt") -> (x = y?=w164:bool)
                    n140 = case shown="真" w164 {
                      tunnel: w163 -> [_ w171]
                      tunnel: w162 -> [_ w170]
                      frame False {
                      }
                      frame True {
                        n141 = flat-sequence {
                          tunnel: w171 -> [w186]
                          tunnel: w170 -> [w175]
                          frame #0 {
                            n142 = call-poly <vilib>:"Read From Spreadsheet File.vi"("transpose (no:F)"=TRUE, "file path (dialog if empty)"=w186) -> ("first row"=w172:dbl[])  [unwired: 5 in, 4 out]
                            n143 = local read "显示：列表显示内容"() -> (w176:string[])
                            n144 = local read "设置：幅度谱总道数"() -> (w181:u32)
                            n145 = Replace Array Subset(array=w176, new element=w175, index=0 ("索引")) -> (w173:string[])
                            n146 = local write "显示：列表显示内容"(w173) -> ()
                            n147 = local write "变量：原始数据"(w172) -> ()
                            n148 = Array Max & Min(array=w172) -> (max value=w180:dbl)  [unwired: 3 out]
                            n149 = Initialize Array(nan ("元素"), w181) -> (w184:dbl[])
                            n150 = Build Array(w172, w184) -> (w185:dbl[][])
                            n151 = Multiply(x=w180, y=1.1) -> (x*y=w178:dbl)
                            n152 = local write "显示：波形图"(w185) -> ()
                            n153 = local write "显示：波形图_预览"(w185) -> ()
                            n154 = local write "变量：图像缓存数组"(w185) -> ()
                            n155 = property on="显示：波形图" class="WFGraph (严格)"("YScale.Maximum"=w178, "YScale.Minimum"=0.0 ("Y标尺.范围:最小值")) -> ()  [unwired: 2 in, 2 out]
                            n156 = property on="显示：波形图_预览" class="WFGraph (严格)"("YScale.Maximum"=w178, "YScale.Minimum"=0.0 ("Y标尺.范围:最小值")) -> ()  [unwired: 2 in, 2 out]
                          }
                          frame #1 {
                            w193 = T5 {"X"=0.0, "Y"=0.0} ("游标.游标位置")
                            n157 = local read "设置：幅度谱总道数"() -> (w194:u32)
                            n158 = property on="显示：波形图_预览" class="WFGraph (严格)"("Cursor.Cursor Position"=w193, "XScale.Maximum"=w194, "XScale.Minimum"=0.0 ("X标尺.范围:最小值")) -> ()  [unwired: 2 in, 2 out]
                            n159 = property on="显示：波形图" class="WFGraph (严格)"("XScale.Maximum"=w194, "XScale.Minimum"=0.0 ("X标尺.范围:最小值"), "Cursor.Cursor Position"=w193, "ActPaletteTool"=0 ("选板:活动工具"), "Plot.Visible?"=TRUE ("曲线.可见"), "Active Plot"=u32 1 ("活动曲线")) -> ()  [unwired: 2 in, 2 out]
                          }
                        }
                      }
                    }
                  }
                  frame True {
                    n160 = flat-sequence {
                      tunnel: w195 -> [w198]
                      frame #0 {
                        n161 = TDMS Open(5:FALSE ("创建索引文件？(T)"), 10:T7."open" ("操作(0:open)"), 11:w198) -> (0:w205:errorcluster, 3:w215:refnum<k34>)  [unwired: 4 in]
                        n162 = TDMS Read(0:w215, 5:"文件属性" ("组名称输入"), 11:w205, 12:string[][] []) -> (4:w209:refnum<k34>, 10:w213:string[][], 15:w204:errorcluster)  [unwired: 4 in, 3 out]
                        n163 = Index Array(array=w213, index (row)=1 ("索引")) -> (element=w211:string[])  [unwired: 1 in]
                        n164 = local write "显示：列表显示内容"(w211) -> ()
                        n165 = TDMS Read(0:w209, 5:"数据" ("组名称输入"), 11:w204, 12:dbl[] []) -> (4:w206:refnum<k34>, 10:w197:dbl[], 15:w203:errorcluster)  [unwired: 4 in, 3 out]
                        n166 = local read "设置：幅度谱总道数"() -> (w202:u32)
                        n167 = TDMS Close(8:w203, 11:w206) -> ()  [unwired: 2 out]
                        n168 = case shown="1024, 默认" w202 {
                          tunnel: w197 -> [w223 w227 w231 w251]
                          tunnel: [w223 w224 w234 w248] -> w196
                          frame 8192 {
                          }
                          frame 4096 {
                            n169 = Decimate 1D Array(w227) -> (w225:dbl[], w226:dbl[])
                            n170 = for {
                              tunnel: w226 -> [w229] mode=indexing
                              tunnel: w225 -> [w230] mode=indexing
                              tunnel: [w228] -> w224 mode=indexing
                              n171 = Add(x=w230, y=w229) -> (x+y=w228:dbl)
                            }
                          }
                          frame 2048 {
                            n172 = Decimate 1D Array(w231) -> (w235:dbl[], w236:dbl[], w233:dbl[], w232:dbl[])
                            n173 = for {
                              tunnel: w236 -> [w240] mode=indexing
                              tunnel: w235 -> [w241] mode=indexing
                              tunnel: [w239] -> w234 mode=indexing
                              tunnel: w233 -> [w238] mode=indexing
                              tunnel: w232 -> [w237] mode=indexing
                              n174 = Compound Arithmetic op=ADD(w241, w240, w238, w237) -> (w239:dbl)
                            }
                          }
                          frame 1024, Default {
                            n175 = Decimate 1D Array(w251) -> (w249:dbl[], w250:dbl[], w247:dbl[], w246:dbl[], w245:dbl[], w244:dbl[], w243:dbl[], w242:dbl[])
                            n176 = for {
                              tunnel: w250 -> [w259] mode=indexing
                              tunnel: w249 -> [w260] mode=indexing
                              tunnel: [w258] -> w248 mode=indexing
                              tunnel: w247 -> [w257] mode=indexing
                              tunnel: w246 -> [w256] mode=indexing
                              tunnel: w245 -> [w255] mode=indexing
                              tunnel: w244 -> [w254] mode=indexing
                              tunnel: w243 -> [w253] mode=indexing
                              tunnel: w242 -> [w252] mode=indexing
                              n177 = Compound Arithmetic op=ADD(w260, w259, w257, w256, w255, w254, w253, w252) -> (w258:dbl)
                            }
                          }
                        }
                        "变量：原始数据" <- w196
                        n178 = Array Max & Min(array=w196) -> (max value=w201:dbl)  [unwired: 3 out]
                        n179 = Initialize Array(nan ("元素"), w202) -> (w221:dbl[])
                        n180 = Build Array(w196, w221) -> (w222:dbl[][])
                        n181 = Multiply(x=w201, y=1.1) -> (x*y=w199:dbl)
                        n182 = local write "显示：波形图"(w222) -> ()
                        n183 = local write "显示：波形图_预览"(w222) -> ()
                        n184 = local write "变量：图像缓存数组"(w222) -> ()
                        n185 = property on="显示：波形图" class="WFGraph (严格)"("YScale.Maximum"=w199, "YScale.Minimum"=0.0 ("Y标尺.范围:最小值")) -> ()  [unwired: 2 in, 2 out]
                        n186 = property on="显示：波形图_预览" class="WFGraph (严格)"("YScale.Maximum"=w199, "YScale.Minimum"=0.0 ("Y标尺.范围:最小值")) -> ()  [unwired: 2 in, 2 out]
                      }
                      frame #1 {
                        w263 = T5 {"X"=0.0, "Y"=0.0} ("游标.游标位置")
                        n187 = local read "设置：幅度谱总道数"() -> (w262:u32)
                        n188 = property on="显示：波形图_预览" class="WFGraph (严格)"("Cursor.Cursor Position"=w263, "XScale.Maximum"=w262, "XScale.Minimum"=0.0 ("X标尺.范围:最小值")) -> ()  [unwired: 2 in, 2 out]
                        n189 = property on="显示：波形图" class="WFGraph (严格)"("XScale.Maximum"=w262, "XScale.Minimum"=0.0 ("X标尺.范围:最小值"), "Cursor.Cursor Position"=w263, "ActPaletteTool"=0 ("选板:活动工具"), "Cursor.Cursor Plot"=0 ("游标.游标关联曲线"), "Active Plot"=u32 1 ("活动曲线"), "Plot.Visible?"=TRUE ("曲线.可见")) -> ()  [unwired: 2 in, 2 out]
                      }
                    }
                  }
                }
              }
              frame True {
              }
            }
          }
          event "按钮_保存": Value Change {
            n190 = event-data() -> ()  [unwired: 1 in, 6 out]
            n191 = call "MCA_SaveDialog.vi"() -> ("保存数据文件至： 2"=w270:path, "数据文件名称： 2"=w269:string, "是否取消？"=w271:bool)  [unwired: 9 in]
            n192 = case shown="假" w271 {
              tunnel: w270 -> [w301 _]
              tunnel: w269 -> [w302 _]
              frame False {
                n193 = local read "显示：列表显示内容"() -> (w295:string[])
                n194 = Strip Path(path=w301) -> (stripped path=w274:path)  [unwired: 1 out]
                n195 = property on="列表框" class="MCListbox (严格)"() -> ("ItemNames"=w293:string[][])  [unwired: 2 in, 2 out]
                n196 = Concatenate Strings(w302, ".txt" ("字符串")) -> (w275:string)
                n197 = TDMS Open(5:FALSE ("创建索引文件？(T)"), 10:T7."create or replace" ("操作(0:open)"), 11:w301) -> (0:w285:errorcluster, 3:w296:refnum<k34>)  [unwired: 4 in]
                n198 = Index Array(array=w293, index (col)=0 ("禁用的索引 (列)")) -> (element=w291:string[])  [unwired: 1 in]
                n199 = Replace Array Subset(array=w295, new element=w302, index=0 ("索引")) -> (w290:string[])
                n200 = Build Path(base path=w274, name or relative path=w275) -> (appended path=w273:path)
                n201 = local write "显示：列表显示内容"(w290) -> ()
                n202 = Build Array(w291, w290) -> (w282:string[][])
                n203 = local read "变量：图像缓存数组"() -> (w280:dbl[][])
                n204 = local read "变量：上次测量原始数据"() -> (w281:dbl[])
                n205 = TDMS Write(0:w296, 5:"文件属性" ("组名称输入（无标题）"), 7:string[] ["属性名称", "值"] ("通道名输入（无标题）"), 9:w282, 11:w285) -> (4:w289:refnum<k34>, 15:w284:errorcluster)  [unwired: 1 in, 2 out]
                n206 = Index Array(array=w280, index (row)=0 ("索引 (行)")) -> (element=w278:dbl[])  [unwired: 1 in]
                n207 = TDMS Write(0:w289, 5:"数据" ("组名称输入（无标题）"), 7:"计数", 9:w281, 11:w284) -> (4:w286:refnum<k34>, 15:w283:errorcluster)  [unwired: 1 in, 2 out]
                n208 = call-poly <vilib>:"Write To Spreadsheet File.vi"("transpose? (no:F)"=TRUE, "1D data"=w278, "file path (dialog if empty)"=w273) -> ()  [unwired: 5 in, 1 out]
                n209 = TDMS Close(8:w283, 11:w286) -> ()  [unwired: 2 out]
              }
              frame True {
              }
            }
          }
          event "按钮_设置": Value Change {
            n210 = event-data() -> ()  [unwired: 1 in, 1 out]
            n211 = local read "设置：信号极性（正T）"() -> (w321:bool)
            n212 = local read "设置：幅度谱总道数"() -> (w322:u32)
            n213 = local read "设置：寻峰灵敏度"() -> (w313:i32)
            n214 = local read "设置：甄别前阈值"() -> (w312:u16)
            n215 = local read "设置：甄别后阈值"() -> (w311:u16)
            n216 = local read "设置：测量时间"() -> (w318:u16)
            n217 = local read "设置：刷新频率"() -> (w317:u16)
            n218 = local read "设置 ： 修正文件路径"() -> (w316:path)
            n219 = case shown="1024, 默认" w322 {
              tunnel: [enum32{"1024", "2048", "4096", "8192"}."1024" ("道数") enum32{"1024", "2048", "4096", "8192"}."2048" ("道数") enum32{"1024", "2048", "4096", "8192"}."4096" ("道数") enum32{"1024", "2048", "4096", "8192"}."8192" ("道数")] -> w315
              frame 1024, Default {
              }
              frame 2048 {
              }
              frame 4096 {
              }
              frame 8192 {
              }
            }
            n220 = Select(t=enum32{"正", "负"}."正" ("y"), s=w321, f=enum32{"正", "负"}."负" ("y")) -> (s? t:f=w314:enum32{"正", "负"})
            n221 = call "MCA_ConfigDialog.vi"("测量最多花费的时间（秒）："=w318, "测量数据刷新频率（个/次）："=w317, "数据文件路径"=w316, "道数"=w315, "输入信号的极性："=w314, "寻峰灵敏度："=w313, "甄别前阈值"=w312, "甄别后阈值"=w311) -> ("输入信号极性"=w310:bool, "甄别后阈值 2"=w308:dbl, "甄别前阈值 2"=w309:dbl, "是否取消？"=w323:bool, "道数最大值"=w307:i32, "数据文件路径 2"=w306:path, "寻峰灵敏度： 2"=w305:u32, "测量数据刷新时间（个/次）： 2"=w304:u32, "测量最多花费的时间（秒）： 2"=w303:u32)  [unwired: 11 in]
            n222 = case shown="假" w323 {
              tunnel: w309 -> [w380 _]
              tunnel: w306 -> [w378 _]
              tunnel: w307 -> [w355 _]
              tunnel: w322 -> [w356 _]
              tunnel: w310 -> [w334 _]
              tunnel: w308 -> [w332 _]
              tunnel: w305 -> [w331 _]
              tunnel: w304 -> [w330 _]
              tunnel: w303 -> [w329 _]
              frame False {
                n223 = Divide(x=w356, y=w355) -> (x/y=w348:dbl)
                n224 = local read "变量：感兴区起点道址"() -> (w354:dbl)
                n225 = local read "变量：感兴区终点道址"() -> (w353:dbl)
                n226 = property on="显示：波形图" class="WFGraph (严格)"("XScale.Maximum"=w355, "XScale.Minimum"=0.0 ("X标尺.范围:最小值")) -> ()  [unwired: 2 in, 2 out]
                n227 = Equal?(x=w378, y=path "") -> (x = y?=w377:bool)
                n228 = property on="显示：波形图_预览" class="WFGraph (严格)"("XScale.Maximum"=w355, "XScale.Minimum"=0.0 ("X标尺.范围:最小值")) -> ()  [unwired: 2 in, 2 out]
                n229 = local write "设置：幅度谱总道数"(w355) -> ()
                n230 = local write "设置：信号极性（正T）"(w334) -> ()
                n231 = local write "设置：甄别后阈值"(w332) -> ()
                n232 = local write "设置：甄别前阈值"(w380) -> ()
                n233 = case shown="真" w377 {
                  tunnel: w378 -> [w441 _]
                  tunnel: [w439 w442] -> w344
                  frame False {
                    n234 = call-poly <vilib>:"Read From Spreadsheet File.vi"("transpose (no:F)"=TRUE, "file path (dialog if empty)"=w441) -> ("first row"=w439:dbl[])  [unwired: 5 in, 4 out]
                  }
                  frame True {
                    n235 = local read "MCA道宽修正数组"() -> (w442:ext[])
                  }
                }
                n236 = local write "设置：寻峰灵敏度"(w331) -> ()
                n237 = local write "设置：刷新频率"(w330) -> ()
                n238 = local write "设置：测量时间"(w329) -> ()
                n239 = local write "变量：每次测量计划用时"(w329) -> ()
                n240 = Divide(x=w354, y=w348) -> (x/y=w352:dbl)
                n241 = Divide(x=w353, y=w348) -> (x/y=w351:dbl)
                n242 = property on="显示：波形图" class="WFGraph (严格)"("Active Cursor"=u32 0 ("活动游标")) -> ("Cursor.Cursor X"=w349:dbl)  [unwired: 2 in, 2 out]
                n243 = local write "变量：感兴区起点道址"(w352) -> ()
                n244 = local write "变量：感兴区终点道址"(w351) -> ()
                n245 = local write "MCA道宽修正数组"(w344) -> ()
                n246 = Divide(x=w349, y=w348) -> (x/y=w347:dbl)
                n247 = local read "变量：原始数据"() -> (w333:dbl[])
                n248 = Divide(x=8192.0, y=w355) -> (x/y=w357:dbl)
                n249 = property on="显示：波形图" class="WFGraph (严格)"("Cursor.Cursor X"=w347) -> ()  [unwired: 2 in, 2 out]
                n250 = property on="显示：波形图_预览" class="WFGraph (严格)"("Cursor.Cursor X"=w347) -> ()  [unwired: 2 in, 2 out]
                n251 = local read "设置：寻峰灵敏度"() -> (w361:i32)
                n252 = local read "设置：信号极性（正T）"() -> (w343:bool)
                n253 = local read "设置：幅度谱总道数"() -> (w340:u32)
                n254 = local read "设置：测量时间"() -> (w365:u16)
                n255 = local read "设置：刷新频率"() -> (w364:u16)
                n256 = local read "设置：甄别前阈值"() -> (w363:u16)
                n257 = local read "设置：甄别后阈值"() -> (w362:u16)
                n258 = stacked-sequence {
                  tunnel: w333 -> [w386 _]
                  tunnel: w357 -> [w385 _]
                  frame #0 {
                    n259 = case shown="8" w385 {
                      tunnel: w386 -> [w389 w393 w402 w417]
                      tunnel: [w389 w390 w399 w414] -> w383
                      frame 1, Default {
                      }
                      frame 2 {
                        n260 = Decimate 1D Array(w393) -> (w391:dbl[], w392:dbl[])
                        n261 = for {
                          tunnel: w392 -> [w395] mode=indexing
                          tunnel: w391 -> [w396] mode=indexing
                          tunnel: [w394] -> w390 mode=indexing
                          n262 = Add(x=w396, y=w395) -> (x+y=w394:dbl)
                        }
                      }
                      frame 4 {
                        n263 = Decimate 1D Array(w402) -> (w400:dbl[], w401:dbl[], w398:dbl[], w397:dbl[])
                        n264 = for {
                          tunnel: w401 -> [w406] mode=indexing
                          tunnel: w400 -> [w407] mode=indexing
                          tunnel: [w405] -> w399 mode=indexing
                          tunnel: w398 -> [w404] mode=indexing
                          tunnel: w397 -> [w403] mode=indexing
                          n265 = Compound Arithmetic op=ADD(w407, w406, w404, w403) -> (w405:dbl)
                        }
                      }
                      frame 8 {
                        n266 = Decimate 1D Array(w417) -> (w415:dbl[], w416:dbl[], w413:dbl[], w412:dbl[], w411:dbl[], w410:dbl[], w409:dbl[], w408:dbl[])
                        n267 = for {
                          tunnel: w416 -> [w425] mode=indexing
                          tunnel: w415 -> [w426] mode=indexing
                          tunnel: [w424] -> w414 mode=indexing
                          tunnel: w413 -> [w423] mode=indexing
                          tunnel: w412 -> [w422] mode=indexing
                          tunnel: w411 -> [w421] mode=indexing
                          tunnel: w410 -> [w420] mode=indexing
                          tunnel: w409 -> [w419] mode=indexing
                          tunnel: w408 -> [w418] mode=indexing
                          n268 = Compound Arithmetic op=ADD(w426, w425, w423, w422, w421, w420, w419, w418) -> (w424:dbl)
                        }
                      }
                    }
                    n269 = for {
                      tunnel: w383 -> [_] mode=indexing
                      tunnel: [nan] -> w387 mode=indexing
                    }
                    n270 = local write "变量：原始数据"(w383) -> ()
                    n271 = Build Array(w383, w387) -> (w384:dbl[][])
                    n272 = local write "显示：波形图"(w384) -> ()
                    n273 = local write "显示：波形图_预览"(w384) -> ()
                    n274 = local write "变量：图像缓存数组"(w384) -> ()
                  }
                  frame #1 {
                    n275 = local read "变量：图像缓存数组"() -> (w436:dbl[][])
                    n276 = Index Array(array=w436, index (row)=0 ("索引 (行)")) -> (element=w437:dbl[])  [unwired: 1 in]
                    n277 = Array Max & Min(array=w437) -> (max value=w430:dbl)  [unwired: 3 out]
                    n278 = Multiply(x=w430, y=1.1) -> (x*y=w433:dbl)
                    n279 = Less?(x=w433, y=10.0) -> (x < y?=w435:bool)
                    n280 = Select(t=10.0, s=w435, f=w433) -> (s? t:f=w427:dbl)
                    n281 = property on="显示：波形图_预览" class="WFGraph (严格)"("YScale.Maximum"=w427, "YScale.Minimum"=0.0 ("Y标尺.范围:最小值")) -> ()  [unwired: 2 in, 2 out]
                    n282 = property on="显示：波形图" class="WFGraph (严格)"("YScale.Maximum"=w427, "YScale.Minimum"=0.0 ("X标尺.范围:最小值")) -> ()  [unwired: 2 in, 2 out]
                  }
                }
                n283 = case shown="假" w343 {
                  tunnel: ["负" ("字符串") "正" ("字符串")] -> w341
                  frame False {
                  }
                  frame True {
                  }
                }
                n284 = Number To Decimal String(number=w361) -> (decimal integer string=w336:string)  [unwired: 1 in]
                n285 = Number To Decimal String(number=w365) -> (decimal integer string=w369:string)  [unwired: 1 in]
                n286 = Number To Decimal String(number=w364) -> (decimal integer string=w374:string)  [unwired: 1 in]
                n287 = Number To Decimal String(number=w363) -> (decimal integer string=w346:string)  [unwired: 1 in]
                n288 = Number To Decimal String(number=w362) -> (decimal integer string=w345:string)  [unwired: 1 in]
                n289 = Number To Decimal String(number=w340) -> (decimal integer string=w338:string)  [unwired: 1 in]
                n290 = Concatenate Strings(w369, "秒" ("字符串")) -> (w370:string)
                n291 = Concatenate Strings(w374, "个/次" ("字符串")) -> (w376:string)
                n292 = local read "显示：列表显示内容"() -> (w367:string[])
                n293 = Replace Array Subset(array=w367, new element #1=w370, index #1=1 ("索引"), new element #2=w376, index #2=2 ("索引"), new element #3=w346, index #3=3 ("索引"), new element #4=w345, index #4=4 ("索引"), new element #5=w341, index #5=5 ("索引"), new element #6=w338, index #6=6 ("索引"), new element #7=w336, index #7=18 ("索引")) -> (w335:string[])
                n294 = local write "显示：列表显示内容"(w335) -> ()
              }
              frame True {
              }
            }
          }
          event "按钮_游标": Value Change {
            # "游标显示时，左右移按钮才可以用才可用"
            n295 = event-data() -> ()  [unwired: 1 in, 1 out]
            n296 = property on="显示：波形图" class="WFGraph (严格)"("Active Cursor"=u32 0 ("活动游标")) -> (error out=w444:errorcluster)  [unwired: 2 in, 1 out]
            n297 = property on="显示：波形图" class="WFGraph (严格)"(error in=w444) -> (error out=w446:errorcluster, "Cursor.Visible"=w454:bool)  [unwired: 1 in, 1 out]
            n298 = property on="显示：波形图_预览" class="WFGraph (严格)"(error in=w444) -> (error out=w445:errorcluster, "Cursor.Visible"=w449:bool)  [unwired: 1 in, 1 out]
            n299 = Not(x=w454) -> (.not. x?=w443:bool)
            n300 = Not(x=w449) -> (.not. x?=w448:bool)
            n301 = property on="显示：波形图" class="WFGraph (严格)"(error in=w446, "Cursor.Visible"=w443) -> ()  [unwired: 1 in, 2 out]
            n302 = property on="显示：波形图_预览" class="WFGraph (严格)"(error in=w445, "Cursor.Visible"=w448) -> ()  [unwired: 1 in, 2 out]
            n303 = Select(t="显示", s=w443, f="隐藏") -> (s? t:f=→"状态栏_游标状态":string)
            n304 = case shown="真" w443 {
              frame False {
                w455 = T6."Disabled and Grayed Out" ("禁用")
                w456 = ""
                n305 = local write "状态栏_游标道址"(w456) -> ()
                n306 = local write "状态栏_游标计数"(w456) -> ()
                n307 = property on="按钮_右移" class="Bool"("DisabledEnum"=w455) -> ()  [unwired: 2 in, 2 out]
                n308 = property on="按钮_左移" class="Bool"("DisabledEnum"=w455) -> ()  [unwired: 2 in, 2 out]
              }
              frame True {
                w459 = T6."Enabled" ("禁用")
                n309 = property on="显示：波形图" class="WFGraph (严格)"() -> (error out=w458:errorcluster, "Cursor.Cursor X"=w465:dbl)  [unwired: 2 in, 1 out]
                n310 = Number To Decimal String(number=w465) -> (decimal integer string=w466:string)  [unwired: 1 in]
                n311 = local write "状态栏_游标道址"(w466) -> ()
                n312 = property on="显示：波形图" class="WFGraph (严格)"(error in=w458, "Cursor.Cursor Plot"=0 ("游标.游标关联曲线")) -> ("Cursor.Cursor Y"=w461:dbl)  [unwired: 1 in, 2 out]
                n313 = property on="按钮_右移" class="Bool"("DisabledEnum"=w459) -> ()  [unwired: 2 in, 2 out]
                n314 = property on="按钮_左移" class="Bool"("DisabledEnum"=w459) -> ()  [unwired: 2 in, 2 out]
                n315 = Number To Decimal String(number=w461) -> (decimal integer string=w463:string)  [unwired: 1 in]
                n316 = Equal?(x=w463, y="NaN") -> (x = y?=w460:bool)
                n317 = case shown="假" w460 {
                  tunnel: w463 -> [w467 _]
                  tunnel: [w467 "0"] -> w464
                  frame False {
                  }
                  frame True {
                  }
                }
                n318 = local write "状态栏_游标计数"(w464) -> ()
              }
            }
          }
          event "按钮_放大": Value Change {
            w473 = 0
            n319 = event-data() -> ()  [unwired: 1 in, 6 out]
            n320 = local read "变量：感兴区起点道址"() -> (w485:dbl)
            n321 = local read "变量：感兴区终点道址"() -> (w482:dbl)
            n322 = Subtract(x=w485, y=w482) -> (x-y=w474:dbl)
            n323 = Divide(x=w474, y=2.0) -> (x/y=w483:dbl)
            n324 = Add(x=w483, y=w482) -> (x+y=w481:dbl)
            n325 = local read "设置：幅度谱总道数"() -> (w472:u32)
            n326 = Add(x=w474, y=w481) -> (x+y=w480:dbl)
            n327 = Subtract(x=w481, y=w474) -> (x-y=w475:dbl)
            n328 = property on="按钮_放大" class="Bool"("DisabledEnum"=T6."Disabled and Grayed Out" ("禁用")) -> ()  [unwired: 2 in, 2 out]
            n329 = Greater?(x=w473, y=w480) -> (0:w479:bool)
            n330 = Less?(x=w475, y=w472) -> (x < y?=w477:bool)
            n331 = Select(t=w473, s=w479, f=w480) -> (s? t:f=w478:dbl)
            n332 = Select(t=w475, s=w477, f=w472) -> (s? t:f=w476:dbl)
            n333 = To Quad Integer(1:w478) -> (0:w470:i64)
            n334 = To Quad Integer(1:w476) -> (0:w471:i64)
            n335 = property on="显示：波形图" class="WFGraph (严格)"("XScale.Maximum"=w471, "XScale.Minimum"=w470) -> ()  [unwired: 2 in, 2 out]
          }
          event "按钮_还原": Value Change {
            w498 = 0.0 ("变量：起点道址")
            w487 = ""
            # "列表复位"
            # "图像数据复位"
            # "游标起点、终点和标记复位"
            n336 = event-data() -> ()  [unwired: 1 in, 1 out]
            n337 = property on="显示：波形图" class="WFGraph (严格)"("Active Cursor"=u32 1 ("活动游标"), "Cursor.Visible"=FALSE ("游标.可见"), "Cursor.Cursor Plot"=1 ("游标.游标关联曲线"), "Cursor.Cursor Name"="" ("游标.游标名")) -> (error out=w489:errorcluster)  [unwired: 2 in, 1 out]
            n338 = local read "设置：幅度谱总道数"() -> (w503:u32)
            n339 = local read "显示：列表显示内容"() -> (w502:string[])
            n340 = property on="显示：波形图_预览" class="WFGraph (严格)"("Cursor.Cursor Position"=T5 {"X"=0.0, "Y"=0.0} ("游标.游标位置")) -> ()  [unwired: 2 in, 2 out]
            n341 = property on="显示：波形图" class="WFGraph (严格)"(error in=w489, "XScale.Maximum"=w503, "XScale.Minimum"=0.0 ("X标尺.范围:最小值"), "Cursor.Cursor Position"=T5 {"X"=0.0, "Y"=0.0} ("游标.游标位置"), "ActPaletteTool"=0 ("选板:活动工具"), "Cursor.Cursor Plot"=0 ("游标.游标关联曲线")) -> ()  [unwired: 1 in, 2 out]
            n342 = Replace Array Subset(array=w502, new element #1=w487, index #1=12 ("索引"), new element #2=w487, index #2=13 ("索引"), new element #3=w487, index #3=14 ("索引"), new element #4=w487, index #4=15 ("索引"), new element #5=w487, index #5=16 ("索引"), new element #6=w487, index #6=17 ("索引")) -> (w501:string[])
            n343 = local write "显示：列表显示内容"(w501) -> ()
            n344 = local read "变量：图像缓存数组"() -> (w488:dbl[][])
            n345 = local write "变量：感兴区起点道址"(w498) -> ()
            n346 = local write "变量：感兴区终点道址"(w498) -> ()
            n347 = local write "显示：波形图_预览"(w488) -> ()
            n348 = local write "显示：波形图"(w488) -> ()
          }
          event "按钮_左移": Value Change {
            n349 = event-data() -> ()  [unwired: 1 in, 6 out]
            n350 = property on="显示：波形图" class="WFGraph (严格)"("Active Cursor"=u32 0 ("活动游标")) -> ("Cursor.Cursor X"=w510:dbl)  [unwired: 2 in, 2 out]
            n351 = property on="显示：波形图" class="WFGraph (严格)"() -> ("XScale.Minimum"=w512:dbl)  [unwired: 2 in, 2 out]
            n352 = Decrement(x=w510) -> (x-1=w513:dbl)
            n353 = Greater?(x=w513, y=w512) -> (0:w514:bool)
            n354 = case shown="真" w514 {
              tunnel: w513 -> [_ w516]
              frame False {
              }
              frame True {
                n355 = property on="显示：波形图" class="WFGraph (严格)"("Cursor.Cursor X"=w516) -> ()  [unwired: 2 in, 2 out]
              }
            }
          }
          event "显示：波形图": Mouse Down {
            # "解决“标记后出现上一次寻峰的结果”的问题"
            n356 = event-data() -> ()  [unwired: 1 in, 8 out]
            n357 = property on="显示：波形图" class="WFGraph (严格)"("Active Cursor"=u32 0 ("活动游标")) -> (error out=w519:errorcluster, "Cursor.Cursor X"=w518:dbl)  [unwired: 2 in, 1 out]
            n358 = property on="显示：波形图" class="WFGraph (严格)"(error in=w519, "Active Cursor"=u32 1 ("活动游标"), "Cursor.Cursor X"=0.0 ("游标.游标位置:游标X坐标"), "Cursor.Cursor Name"="" ("游标.游标名")) -> ()  [unwired: 1 in, 2 out]
            n359 = local write "变量：感兴区起点道址"(w518) -> ()
          }
          event "显示：波形图": Mouse Up {
            n360 = event-data() -> ()  [unwired: 1 in, 8 out]
            n361 = flat-sequence {
              frame #0 {
                n362 = property on="显示：波形图" class="WFGraph (严格)"("Active Cursor"=u32 0 ("活动游标")) -> ("Cursor.Cursor X"=w525:dbl)  [unwired: 2 in, 2 out]
                n363 = local write "变量：感兴区终点道址"(w525) -> ()
              }
              frame #1 {
                n364 = local read "变量：感兴区起点道址"() -> (w529:dbl)
                n365 = local read "变量：感兴区终点道址"() -> (w528:dbl)
                n366 = Equal?(x=w529, y=w528) -> (x = y?=w527:bool)
                n367 = case shown="假" w527 {
                  tunnel: w528 -> [w534 _]
                  tunnel: w529 -> [w535 _]
                  frame False {
                    # "若起点比终点大，起点和中间交换"
                    n368 = local read "状态：停止变量"() -> (w531:bool)
                    n369 = Greater?(x=w535, y=w534) -> (0:w536:bool)
                    n370 = case shown="假" w536 {
                      tunnel: w535 -> [w539 w541]
                      tunnel: w534 -> [w538 w540]
                      tunnel: [w539 w540] -> w533
                      tunnel: [w538 w541] -> w532
                      frame False {
                        # "起点比终点小，不变"
                      }
                      frame True {
                      }
                    }
                    n371 = case shown="真" w531 {
                      frame False {
                      }
                      frame True {
                        n372 = property on="按钮_寻峰" class="Bool"("DisabledEnum"=T6."Enabled" ("禁用")) -> ()  [unwired: 2 in, 2 out]
                      }
                    }
                    n373 = local write "变量：感兴区起点道址"(w533) -> ()
                    n374 = local write "变量：感兴区终点道址"(w532) -> ()
                    n375 = property on="按钮_放大" class="Bool"("DisabledEnum"=T6."Enabled" ("禁用")) -> ()  [unwired: 2 in, 2 out]
                  }
                  frame True {
                  }
                }
              }
            }
          }
          event "按钮_右移": Value Change {
            n376 = event-data() -> ()  [unwired: 1 in, 6 out]
            n377 = property on="显示：波形图" class="WFGraph (严格)"("Active Cursor"=u32 0 ("活动游标")) -> ("Cursor.Cursor X"=w542:dbl)  [unwired: 2 in, 2 out]
            n378 = property on="显示：波形图" class="WFGraph (严格)"() -> ("XScale.Maximum"=w544:dbl)  [unwired: 2 in, 2 out]
            n379 = Increment(x=w542) -> (x+1=w545:dbl)
            n380 = Less Or Equal?(x=w545, y=w544) -> (x <= y?=w546:bool)
            n381 = case shown="真" w546 {
              tunnel: w545 -> [_ w548]
              frame False {
              }
              frame True {
                n382 = property on="显示：波形图" class="WFGraph (严格)"("Cursor.Cursor X"=w548) -> ()  [unwired: 2 in, 2 out]
              }
            }
          }
          event Value Change {
            n383 = event-data() -> ()  [unwired: 1 in, 1 out]
            n384 = stacked-sequence {
              frame #0 {
                n385 = local read "变量：感兴区起点道址"() -> (w565:dbl)
                n386 = local read "变量：感兴区终点道址"() -> (w564:dbl)
                n387 = local read "变量：图像缓存数组"() -> (w563:dbl[][])
                n388 = call "MCA_Confirming Interested area Dialog.vi"("终点道址："=w564, "起点道址："=w565) -> ("终点道址： 2"=w553:u32, "起点道址： 2"=w555:u32)
                n389 = Index Array(array=w563, index (row)=0 ("索引 (行)")) -> (element=w560:dbl[])  [unwired: 1 in]
                n390 = call "一线双色计算.vi"("输入一维数组"=w560, "right corsor"=w553, "left corsor"=w555) -> ("输出波形数组"=w562:dbl[][])
                n391 = local write "变量：感兴区终点道址"(w553) -> ()
                n392 = local write "显示：波形图_预览"(w562) -> ()
                n393 = local write "显示：波形图"(w562) -> ()
                n394 = local write "变量：感兴区起点道址"(w555) -> ()
                n395 = local read "显示：列表显示内容"() -> (w558:string[])
                n396 = Number To Fractional String(number=w553, precision (6)=i16 0 ("精度(6)")) -> (F-format string=w552:string)  [unwired: 2 in]
                n397 = Number To Fractional String(number=w555, precision (6)=i16 0 ("精度(6)")) -> (F-format string=w554:string)  [unwired: 2 in]
                n398 = Replace Array Subset(array=w558, new element #1=w554, index #1=12 ("索引"), new element #2=w552, index #2=13 ("索引")) -> (w559:string[])
                n399 = local write "显示：列表显示内容"(w559) -> ()
              }
              frame #1 {
                n400 = local read "变量：图像缓存数组"() -> (w616:dbl[][])
                n401 = property on="按钮_寻峰" class="Bool"("DisabledEnum"=T6."Disabled and Grayed Out" ("禁用")) -> ()  [unwired: 2 in, 2 out]
                n402 = local read "变量：感兴区起点道址"() -> (w614:dbl)
                n403 = local read "变量：感兴区终点道址"() -> (w613:dbl)
                n404 = Index Array(array=w616, index (row)=0 ("索引 (行)")) -> (element=w612:dbl[])  [unwired: 1 in]
                n405 = for {
                  tunnel: w612 -> [w621] mode=indexing
                  tunnel: w614 -> [w626]
                  tunnel: w613 -> [w619]
                  tunnel: [w620] -> w575 mode=indexing
                  tunnel: [w618] -> w576 mode=indexing
                  i -> [w618]
                  n406 = Greater Or Equal?(x=w618, y=w626) -> (x >= y?=w625:bool)
                  n407 = Less Or Equal?(x=w618, y=w619) -> (x <= y?=w624:bool)
                  n408 = And(x=w625, y=w624) -> (x .and. y?=w623:bool)
                  n409 = Select(t=w621, s=w623, f=0.0) -> (s? t:f=w620:dbl)
                }
                n410 = Array Max & Min(array=w575) -> (max value=w583:dbl)  [unwired: 3 out]
                n411 = Multiply(x=w583, y=0.85) -> (x*y=w584:dbl)
                n412 = call <vilib>:"Gaussian Peak Fit.vi"("Y"=w575, "X"=w576) -> ("center"=→"center":dbl, "standard deviation"=w573:dbl)  [unwired: 7 in, 5 out]
                n413 = call <vilib>:"Peak Detector.vi"("peaks/valleys"=enum32{"Peaks", "Valleys"}."Peaks", "width"="设置：寻峰灵敏度", "threshold"=w584, "X"=w575) -> ("Amplitudes"=w578:dbl[], "Locations"=w581:dbl[])  [unwired: 3 in, 3 out]
                n414 = Multiply(x=2.355, y=w573) -> (x*y=w568:dbl)
                "结果：半高宽" <- w568
                n415 = Index Array(array=w581, index=0 ("索引")) -> (element=w569:dbl)
                "结果：峰位" <- w569
                n416 = Index Array(array=w578, index=0 ("索引")) -> ()  [unwired: 1 out]
                n417 = Add Array Elements(numeric array=w575) -> (sum=w566:dbl)
                "结果：净面积" <- w566
                n418 = Divide(x=w568, y=w569) -> (x/y=w593:dbl)
                n419 = Equal?(x=w569, y=0.0) -> (x = y?=w571:bool)
                n420 = Multiply(x=w593, y=100.0) -> (x*y=w591:dbl)
                n421 = Number To Fractional String(number=w569, precision (6)=i16 2 ("精度(6)")) -> (F-format string=w570:string)  [unwired: 2 in]
                n422 = Number To Fractional String(number=w568, precision (6)=i16 2 ("精度(6)")) -> (F-format string=w598:string)  [unwired: 2 in]
                n423 = Number To Fractional String(number=w566, precision (6)=i16 0 ("精度(6)")) -> (F-format string=w595:string)  [unwired: 2 in]
                n424 = local read "显示：列表显示内容"() -> (w602:string[])
                n425 = case shown="真" w571 {
                  frame False {
                  }
                  frame True {
                    n426 = One Button Dialog(message="    未寻到有效峰值！请设置合适的寻峰灵敏度后，重新寻峰！    \n（寻峰灵敏度请按工具栏“设置”按钮，“寻峰设置”标签设置）" ("消息")) -> ()  [unwired: 1 in, 1 out]
                  }
                }
                n427 = Number To Fractional String(number=w591, precision (6)=i16 2 ("精度(6)")) -> (F-format string=w589:string)  [unwired: 2 in]
                n428 = Number To Fractional String(number=w569, precision (6)=i16 2 ("精度(6)")) -> (F-format string=w606:string)  [unwired: 2 in]
                n429 = Concatenate Strings(w589, "%" ("字符串")) -> (w587:string)
                n430 = property on="显示：波形图" class="WFGraph (严格)"("Active Cursor"=u32 1 ("活动游标"), "Cursor.Cursor X"=w569, "Cursor.Visible"=TRUE ("游标.可见"), "Cursor.Cursor Plot"=1 ("游标.游标关联曲线"), "Cursor.Cursor Name"=w606) -> (error out=w608:errorcluster)  [unwired: 2 in, 1 out]
                n431 = Replace Array Subset(array=w602, new element #1=w570, index #1=14 ("索引"), new element #2=w598, index #2=15 ("索引"), new element #3=w595, index #3=16 ("索引"), new element #4=w587, index #4=17 ("索引")) -> (w601:string[])
                n432 = local write "显示：列表显示内容"(w601) -> ()
                n433 = property on="显示：波形图" class="WFGraph (严格)"(error in=w608, "Active Cursor"=u32 0 ("活动游标")) -> ()  [unwired: 1 in, 2 out]
              }
            }
          }
          event Key Down {
            n434 = event-data() -> ("VKey"=w627:T8)  [unwired: 1 in, 5 out]
            n435 = case shown="\"Right\"" w627 {
              frame "Left" {
                n436 = property on="显示：波形图" class="WFGraph (严格)"() -> ("Cursor.Visible"=w629:bool)  [unwired: 2 in, 2 out]
                n437 = case shown="真" w629 {
                  frame False {
                  }
                  frame True {
                    n438 = property on="显示：波形图" class="WFGraph (严格)"("Active Cursor"=u32 0 ("活动游标")) -> (error out=w630:errorcluster, "Cursor.Cursor X"=w631:dbl)  [unwired: 2 in, 1 out]
                    n439 = property on="显示：波形图" class="WFGraph (严格)"() -> ("XScale.Minimum"=w633:dbl)  [unwired: 2 in, 2 out]
                    n440 = Decrement(x=w631) -> (x-1=w634:dbl)
                    n441 = Greater?(x=w634, y=w633) -> (0:w635:bool)
                    n442 = case shown="真" w635 {
                      tunnel: w634 -> [_ w636]
                      tunnel: w630 -> [_ _]
                      frame False {
                      }
                      frame True {
                        n443 = property on="显示：波形图" class="WFGraph (严格)"("Cursor.Cursor X"=w636) -> ()  [unwired: 2 in, 2 out]
                      }
                    }
                  }
                }
              }
              frame "Right" {
                n444 = property on="显示：波形图" class="WFGraph (严格)"() -> ("Cursor.Visible"=w637:bool)  [unwired: 2 in, 2 out]
                n445 = case shown="真" w637 {
                  frame False {
                  }
                  frame True {
                    n446 = property on="显示：波形图" class="WFGraph (严格)"("Active Cursor"=u32 0 ("活动游标")) -> (error out=w638:errorcluster, "Cursor.Cursor X"=w639:dbl)  [unwired: 2 in, 1 out]
                    n447 = property on="显示：波形图" class="WFGraph (严格)"() -> ("XScale.Maximum"=w641:dbl)  [unwired: 2 in, 2 out]
                    n448 = Increment(x=w639) -> (x+1=w642:dbl)
                    n449 = Less Or Equal?(x=w642, y=w641) -> (x <= y?=w643:bool)
                    n450 = case shown="真" w643 {
                      tunnel: w642 -> [_ w644]
                      tunnel: w638 -> [_ _]
                      frame False {
                      }
                      frame True {
                        n451 = property on="显示：波形图" class="WFGraph (严格)"("Cursor.Cursor X"=w644) -> ()  [unwired: 2 in, 2 out]
                      }
                    }
                  }
                }
              }
              frame "ASCII", Default {
              }
            }
          }
        }
      }
      frame "完成" {
      }
    }
  }
  n452 = while {
    stop <- w647 stop-if-true
    n453 = event shown="[3] \"按钮_开始\": 值改变" {
      selector: _ -> [_ _ _ _]
      dyn-events: _ -> [_ _ _ _]
      timeout: _ -> [_ _ _ _]
      tunnel: [_ _ TRUE _] -> w647
      event Timeout {
        n454 = event-data() -> ()  [unwired: 1 in, 1 out]
      }
      event "按钮_复位": Value Change {
        w669 = 0.0 ("变量：起点道址")
        w653 = 0.0 ("已测量时间")
        w674 = ""
        w661 = T6."Disabled and Grayed Out" ("禁用")
        n455 = event-data() -> ()  [unwired: 1 in, 1 out]
        n456 = local read "变量：每次测量计划用时"() -> (w649:u16)
        n457 = local read "显示：列表显示内容"() -> (w660:string[])
        n458 = property on="显示：波形图" class="WFGraph (严格)"("Active Cursor"=u32 1 ("活动游标"), "Cursor.Visible"=FALSE ("游标.可见"), "Cursor.Cursor Plot"=1 ("游标.游标关联曲线"), "Cursor.Cursor Name"="" ("游标.游标名")) -> ()  [unwired: 2 in, 2 out]
        n459 = Number To Decimal String(number=w649) -> (decimal integer string=w650:string)  [unwired: 1 in]
        n460 = property on="按钮_开始" class="Bool"("DisabledEnum"=T6."Enabled" ("禁用")) -> ()  [unwired: 2 in, 2 out]
        n461 = Concatenate Strings(w650, "秒" ("字符串")) -> (w648:string)
        n462 = Replace Array Subset(array=w660, new element #1="未命名" ("新元素/子数组"), index #1=0 ("索引"), new element #2=w674, index #2=7 ("索引"), new element #3=w674, index #3=8 ("索引"), new element #4=w674, index #4=9 ("索引"), new element #5=w674, index #5=10 ("索引"), new element #6=w674, index #6=11 ("索引"), new element #7=w674, index #7=12 ("索引"), new element #8=w674, index #8=13 ("索引"), new element #9=w674, index #9=14 ("索引"), new element #10=w674, index #10=15 ("索引"), new element #11=w674, index #11=16 ("索引"), new element #12=w674, index #12=17 ("索引"), new element #13=w648, index #13=1 ("索引")) -> (w687:string[])
        n463 = local write "显示：列表显示内容"(w687) -> ()
        n464 = local write "变量 ： 上次测量总计数"(w653) -> ()
        n465 = local write "变量 : 实时总计数"(w653) -> ()
        n466 = local write "状态：已测时间"(w653) -> ()
        n467 = local write "状态：本次测量和上次未完成测量时间和"(w653) -> ()
        n468 = local write "状态：上次未完成测试的已测时间"(w653) -> ()
        n469 = local write "状态：本次测试已测时间"(w653) -> ()
        n470 = local read "变量：每次测量计划用时"() -> (w654:u16)
        n471 = property on="按钮_寻峰" class="Bool"("DisabledEnum"=w661) -> ()  [unwired: 2 in, 2 out]
        n472 = property on="按钮_右移" class="Bool"("DisabledEnum"=w661) -> ()  [unwired: 2 in, 2 out]
        n473 = property on="按钮_左移" class="Bool"("DisabledEnum"=w661) -> ()  [unwired: 2 in, 2 out]
        n474 = property on="按钮_放大" class="Bool"("DisabledEnum"=w661) -> ()  [unwired: 2 in, 2 out]
        n475 = property on="按钮_停止" class="Bool (严格)"("DisabledEnum"=w661) -> ()  [unwired: 2 in, 2 out]
        n476 = local read "设置：幅度谱总道数"() -> (w689:u32)
        n477 = local write "状态栏_计数率"(T3 "" ("状态栏_计数率")) -> ()
        n478 = local write "状态栏_测量状态"(T3 "停止" ("状态栏_测量状态")) -> ()
        n479 = local write "设置：测量时间"(w654) -> ()
        n480 = local write "变量：感兴区起点道址"(w669) -> ()
        n481 = local write "变量：感兴区终点道址"(w669) -> ()
        n482 = property on="显示：波形图" class="WFGraph (严格)"("XScale.Maximum"=w689, "XScale.Minimum"=0.0 ("X标尺.范围:最小值"), "Cursor.Cursor Position"=T5 {"X"=0.0, "Y"=0.0} ("游标.游标位置"), "Active Cursor"=0 ("游标.游标关联曲线")) -> (error out=w691:errorcluster, "Cursor.Visible"=w666:bool)  [unwired: 2 in, 1 out]
        n483 = case shown="真" w666 {
          frame False {
          }
          frame True {
            w700 = "0"
            n484 = local write "状态栏_游标道址"(w700) -> ()
            n485 = local write "状态栏_游标计数"(w700) -> ()
          }
        }
        n486 = Initialize Array(nan ("元素"), 8192 ("维数大小")) -> (w662:dbl[])
        n487 = Initialize Array(0.0 ("元素"), 8192 ("维数大小")) -> (w665:dbl[])
        n488 = Initialize Array(nan ("元素"), 8192 ("维数大小")) -> (w655:dbl[])
        n489 = local write "变量：上次测量原始数据"(w665) -> ()
        n490 = Build Array(w662, w662) -> (w699:dbl[][])
        n491 = property on="显示：波形图_预览" class="WFGraph (严格)"(error in=w691, "XScale.Maximum"=w689, "XScale.Minimum"=0.0 ("X标尺.范围:最小值"), "Cursor.Cursor Position"=T5 {"X"=0.0, "Y"=0.0} ("游标.游标位置")) -> ()  [unwired: 1 in, 2 out]
        n492 = property on="显示：波形图" class="WFGraph (严格)"("YScale.Maximum"=10.0 ("Y标尺.范围:最大值"), "YScale.Minimum"=0.0 ("Y标尺.范围:最大值")) -> ()  [unwired: 2 in, 2 out]
        n493 = local write "变量：原始数据"(w655) -> ()
        n494 = local write "变量：图像缓存数组"(w699) -> ()
        n495 = local write "显示：波形图_预览"(w699) -> ()
        n496 = local write "显示：波形图"(w699) -> ()
        "变量：上次测量时间" <- w653
      }
      event Panel Close; "按钮_退出": Value Change {
        w719 = T3 "" ("状态栏_游标计数")
        n497 = event-data() -> ()  [unwired: 1 in, 3 out]
        n498 = property on="按钮_开始" class="Bool"("DisabledEnum"=T6."Enabled" ("禁用")) -> ()  [unwired: 2 in, 2 out]
        n499 = Initialize Array(nan ("元素"), 8192 ("维数大小")) -> (w730:dbl[])
        n500 = Build Array(w730, w730) -> (w733:dbl[][])
        n501 = local write "变量：图像缓存数组"(w733) -> ()
        n502 = local write "显示：波形图_预览"(w733) -> ()
        n503 = local write "显示：波形图"(w733) -> ()
        n504 = property on="显示：波形图" class="WFGraph (严格)"("Active Cursor"=u32 1 ("活动游标"), "Cursor.Visible"=FALSE ("游标.可见"), "Cursor.Cursor Plot"=1 ("游标.游标关联曲线"), "Cursor.Cursor Name"="" ("游标.游标名")) -> (error out=w711:errorcluster)  [unwired: 2 in, 1 out]
        n505 = property on="按钮_停止" class="Bool (严格)"("DisabledEnum"=T6."Disabled and Grayed Out" ("禁用")) -> ()  [unwired: 2 in, 2 out]
        n506 = property on="显示：波形图" class="WFGraph (严格)"(error in=w711, "Active Cursor"=u32 0 ("活动游标")) -> (error out=w706:errorcluster)  [unwired: 1 in, 1 out]
        n507 = property on="显示：波形图" class="WFGraph (严格)"(error in=w706, "Cursor.Cursor Position"=T5 {"X"=0.0, "Y"=0.0} ("游标.游标位置"), "Cursor.Visible"=FALSE ("游标.可见"), "YScale.Maximum"=10.0 ("Y标尺.范围:最大值"), "YScale.Minimum"=0.0 ("Y标尺.范围:最小值")) -> (error out=w703:errorcluster)  [unwired: 1 in, 1 out]
        n508 = Initialize Array("", 19 ("维数大小")) -> (w724:string[])
        n509 = property on="列表框" class="MCListbox (严格)"() -> ("ItemNames"=w726:string[][])  [unwired: 2 in, 2 out]
        n510 = Replace Array Subset(array=w724, new element="未命名" ("新元素/子数组"), index=0 ("索引")) -> (w715:string[])
        n511 = property on="显示：波形图_预览" class="WFGraph (严格)"(error in=w703, "Cursor.Cursor Position"=T5 {"X"=0.0, "Y"=0.0} ("游标.游标位置"), "Cursor.Visible"=FALSE ("游标.可见")) -> ()  [unwired: 1 in, 2 out]
        n512 = Replace Array Subset(array=w726, new element=w715, index (col)=1 ("禁用的索引 (列)")) -> (w727:string[][])  [unwired: 1 in]
        n513 = property on="列表框" class="MCListbox (严格)"("ItemNames"=w727) -> ()  [unwired: 2 in, 2 out]
        n514 = local write "状态栏_游标状态"(T3 "隐藏" ("状态栏_游标状态")) -> ()
        n515 = local write "状态栏_测量状态"(T3 "停止" ("状态栏_测量状态")) -> ()
        n516 = local write "状态栏_游标计数"(w719) -> ()
        n517 = local write "状态栏_游标道址"(w719) -> ()
        n518 = local write "状态栏_计数率"(T3 "" ("状态栏_计数率")) -> ()
      }
      event "按钮_开始": Value Change {
        n519 = event-data() -> ()  [unwired: 1 in, 1 out]
        n520 = local read "变量：剩余使用时间"() -> (w737:dbl)
        n521 = local read "状态：停止变量"() -> (w739:bool)
        n522 = Greater?(x=w737, y=0.0) -> (0:w735:bool)
        n523 = And(x=w739, y=w735) -> (x .and. y?=w738:bool)
        n524 = case shown="真" w738 {
          frame False {
          }
          frame True {
            n525 = stacked-sequence {
              frame #0 {
                w749 = ""
                w763 = T6."Disabled and Grayed Out" ("禁用")
                n526 = local read "状态：本次测量和上次未完成测量时间和"() -> (w740:dbl)
                n527 = local read "变量：每次测量计划用时"() -> (w742:u16)
                n528 = local write "状态：停止变量"(FALSE ("停止变量")) -> ()
                n529 = local read "设置：信号极性（正T）"() -> (w743:bool)
                n530 = local read "设置：甄别后阈值"() -> (w745:u16)
                n531 = local read "设置：甄别前阈值"() -> (w744:u16)
                n532 = Greater Or Equal?(x=w740, y=w742) -> (x >= y?=w741:bool)
                n533 = case shown="真" w741 {
                  frame False {
                    n534 = local read "状态：本次测试已测时间"() -> (→"状态：上次未完成测试的已测时间":dbl)
                  }
                  frame True {
                    w768 = 0.0 ("状态：上次未完成测试的已测时间")
                    n535 = local read "变量：每次测量计划用时"() -> (w770:u16)
                    n536 = local read "设置：测量时间"() -> (w771:u16)
                    n537 = local write "状态：上次未完成测试的已测时间"(w768) -> ()
                    n538 = local write "状态：本次测量和上次未完成测量时间和"(w768) -> ()
                    n539 = Add(x=w771, y=w770) -> (x+y=w769:u16)
                    n540 = local write "设置：测量时间"(w769) -> ()
                  }
                }
                n541 = call "MCA_init.vi"("下阈值"=w745, "设置：信号极性（正T）"=w743, "上阈值"=w744) -> ()
                n542 = property on="按钮_复位" class="Bool"("DisabledEnum"=T6."Disabled and Grayed Out" ("禁用")) -> ()  [unwired: 2 in, 2 out]
                n543 = property on="按钮_开始" class="Bool"("DisabledEnum"=w763) -> ()  [unwired: 2 in, 2 out]
                n544 = property on="按钮_打开" class="Bool"("DisabledEnum"=w763) -> ()  [unwired: 2 in, 2 out]
                n545 = property on="按钮_保存" class="Bool"("DisabledEnum"=w763) -> ()  [unwired: 2 in, 2 out]
                n546 = property on="按钮_设置" class="Bool"("DisabledEnum"=w763) -> ()  [unwired: 2 in, 2 out]
                n547 = local read "显示：列表显示内容"() -> (w750:string[])
                n548 = Get Date/Time In Seconds() -> (seconds since 1Jan1904=w748:timestamp)
                n549 = Get Date/Time String(date format (0)=enum16{"short", "long", "abbreviated"}."long" ("日期格式(0)"), seconds (now)=w748) -> (date string=w746:string)  [unwired: 1 in, 1 out]
                n550 = property on="按钮_停止" class="Bool (严格)"("DisabledEnum"=T6."Enabled" ("禁用")) -> ()  [unwired: 2 in, 2 out]
                n551 = Replace Array Subset(array=w750, new element #1=w746, index #1=7 ("索引"), new element #2=w749, index #2=8 ("索引"), new element #3=w749, index #3=17 ("索引"), new element #4=w749, index #4=12 ("索引"), new element #5=w749, index #5=13 ("索引"), new element #6=w749, index #6=14 ("索引"), new element #7=w749, index #7=15 ("索引"), new element #8=w749, index #8=16 ("索引")) -> (w752:string[])
                n552 = local write "显示：列表显示内容"(w752) -> ()
                n553 = local write "状态栏_计数率"(T3 "" ("状态栏_计数率")) -> ()
                n554 = local write "状态栏_测量状态"(T3 "正在测量..." ("状态栏_测量状态")) -> ()
                "状态：刷新次数" <- 1
              }
              frame #1 {
                n555 = Tick Count (ms)() -> (millisecond timer value=w772:u32)
                "状态：测量开始时间" <- w772
                n556 = while {
                  tunnel: w772 -> [w774]
                  stop <- w775 stop-if-true
                  n557 = stacked-sequence {
                    tunnel: w774 -> [w779 _ _]
                    frame #0 {
                      n558 = while {
                        tunnel: w779 -> [w790]
                        stop <- w796 stop-if-true
                        n559 = local read "状态：刷新次数"() -> (w803:i32)
                        n560 = local read "设置：刷新频率"() -> (w802:u16)
                        n561 = local read "变量：上次测量时间"() -> (w783:dbl)
                        n562 = Tick Count (ms)() -> (millisecond timer value=w791:u32)
                        n563 = call "MCA_count.vi"() -> ("多道计数"=w780:i32)
                        "变量：实时计数" <- w780
                        n564 = Subtract(x=w791, y=w790) -> (x-y=w793:u32)
                        n565 = Multiply(x=w803, y=w802) -> (x*y=w801:i32)
                        n566 = Divide(x=w793, y=u32 1000) -> (x/y=w781:dbl)
                        n567 = Greater Or Equal?(x=w780, y=w801) -> (x >= y?=w800:bool)
                        n568 = Add(x=w783, y=w781) -> (x+y=w782:dbl)
                        n569 = local read "变量：每次测量计划用时"() -> (w797:u16)
                        n570 = local read "状态：停止变量"() -> (w798:bool)
                        n571 = case shown="真" w800 {
                          tunnel: [FALSE TRUE] -> w799
                          frame False {
                          }
                          frame True {
                            n572 = local read "状态：刷新次数"() -> (w807:i32)
                            n573 = Increment(x=w807) -> (x+1=w806:i32)
                            n574 = local write "状态：刷新次数"(w806) -> ()
                          }
                        }
                        n575 = local read "显示：列表显示内容"() -> (w788:string[])
                        n576 = Number To Decimal String(number=w782) -> (decimal integer string=w786:string)  [unwired: 1 in]
                        n577 = Concatenate Strings(w786, "秒" ("字符串")) -> (w784:string)
                        n578 = Greater Or Equal?(x=w781, y=w797) -> (x >= y?=w794:bool)
                        n579 = Or(x=w799, y=w798) -> (x .or. y?=w795:bool)
                        n580 = Replace Array Subset(array=w788, new element=w784, index=8 ("索引")) -> (w789:string[])
                        n581 = Or(x=w795, y=w794) -> (x .or. y?=w796:bool)
                        n582 = local write "显示：列表显示内容"(w789) -> ()
                      }
                    }
                    frame #1 {
                      # "冗余是为了保证先计算实时计数率，再赋给下次计算的初始值"
                      n583 = local read "变量：实时计数"() -> (w817:i32)
                      n584 = local read "状态：测量开始时间"() -> (w829:u32)
                      n585 = local read "变量 ： 上次测量总计数"() -> (w835:u32)
                      n586 = local read "变量：上次测量时间"() -> (w833:dbl)
                      n587 = Tick Count (ms)() -> (millisecond timer value=w826:u32)
                      n588 = local read "变量 : 实时总计数"() -> (w844:u64)
                      n589 = local read "状态：已测时间"() -> (w836:dbl)
                      n590 = Subtract(x=w826, y=w829) -> (x-y=w828:u32)
                      n591 = Divide(x=w828, y=u32 1000) -> (x/y=w808:dbl)
                      "状态：本次测试已测时间" <- w808
                      n592 = Add(x=w817, y=w835) -> (x+y=w834:u32)
                      n593 = Subtract(x=w817, y=w844) -> (x-y=w842:u64)
                      n594 = local read "状态：上次未完成测试的已测时间"() -> (w810:dbl)
                      n595 = Subtract(x=w808, y=w836) -> (x-y=w840:dbl)
                      n596 = Divide(x=w842, y=w840) -> (x/y=w837:dbl)
                      n597 = Number To Decimal String(number=w837) -> (decimal integer string=w838:string)  [unwired: 1 in]
                      n598 = Add(x=w833, y=w808) -> (x+y=w816:dbl)
                      n599 = local read "状态：已测时间"() -> (w839:dbl)
                      n600 = Add(x=w842, y=w844) -> (x+y=w843:u64)
                      n601 = local write "状态栏_计数率"(w838) -> ()
                      n602 = local write "变量 : 实时总计数"(w843) -> ()
                      n603 = Add(x=w839, y=w840) -> (x+y=w841:dbl)
                      n604 = local write "状态：已测时间"(w841) -> ()
                      n605 = Add(x=w810, y=w808) -> (x+y=→"状态：本次测量和上次未完成测量时间和":dbl)
                      n606 = local read "设置：测量时间"() -> (w811:u16)
                      n607 = Number To Decimal String(number=w834) -> (decimal integer string=w825:string)  [unwired: 1 in]
                      n608 = Divide(x=w834, y=w816) -> (x/y=w831:dbl)
                      n609 = Number To Decimal String(number=w816) -> (decimal integer string=w821:string)  [unwired: 1 in]
                      n610 = Number To Decimal String(number=w831) -> (decimal integer string=w832:string)  [unwired: 1 in]
                      n611 = Number To Decimal String(number=w811) -> (decimal integer string=w815:string)  [unwired: 1 in]
                      n612 = local read "显示：列表显示内容"() -> (w819:string[])
                      n613 = Concatenate Strings(w821, "秒" ("字符串")) -> (w820:string)
                      n614 = Concatenate Strings(w815, "秒" ("字符串")) -> (w812:string)
                      n615 = Replace Array Subset(array=w819, new element #1=w820, index #1=8 ("索引"), new element #2=w825, index #2=10 ("索引"), new element #3=w832, index #3=11 ("索引"), new element #4=w812, index #4=1 ("索引")) -> (w823:string[])
                      n616 = local write "显示：列表显示内容"(w823) -> ()
                    }
                    frame #2 {
                      n617 = local read "变量：上次测量原始数据"() -> (w860:dbl[])
                      n618 = local read "MCA道宽修正数组"() -> (w847:ext[])
                      n619 = local read "设置：幅度谱总道数"() -> (w859:u32)
                      n620 = call "MCA_slave.vi"() -> ("波形图"=w845:i32[])
                      n621 = for {
                        tunnel: w845 -> [w914] mode=indexing
                        tunnel: w860 -> [w915] mode=indexing
                        tunnel: w847 -> [w912] mode=indexing
                        tunnel: [w909] -> w846 mode=indexing
                        n622 = Add(x=w914, y=w915) -> (x+y=w913:dbl)
                        n623 = Multiply(x=w913, y=w912) -> (x*y=w911:ext)
                        n624 = Round To Nearest(number=w911) -> (nearest integer value=w910:ext)
                        n625 = To Unsigned Long Integer(number=w910) -> (unsigned 32bit integer=w909:u32)
                      }
                      n626 = Divide(x=8192.0, y=w859) -> (x/y=w857:dbl)
                      n627 = case shown="8" w857 {
                        tunnel: [w870 w872 w881 w896] -> w848
                        tunnel: w846 -> [w870 w871 w878 w889]
                        frame 1, Default {
                        }
                        frame 2 {
                          n628 = Decimate 1D Array(w871) -> (w873:u32[], w874:u32[])
                          n629 = for {
                            tunnel: w874 -> [w876] mode=indexing
                            tunnel: w873 -> [w877] mode=indexing
                            tunnel: [w875] -> w872 mode=indexing
                            n630 = Add(x=w877, y=w876) -> (x+y=w875:u32)
                          }
                        }
                        frame 4 {
                          n631 = Decimate 1D Array(w878) -> (w882:u32[], w883:u32[], w880:u32[], w879:u32[])
                          n632 = for {
                            tunnel: w883 -> [w887] mode=indexing
                            tunnel: w882 -> [w888] mode=indexing
                            tunnel: [w886] -> w881 mode=indexing
                            tunnel: w880 -> [w885] mode=indexing
                            tunnel: w879 -> [w884] mode=indexing
                            n633 = Compound Arithmetic op=ADD(w888, w887, w885, w884) -> (w886:u32)
                          }
                        }
                        frame 8 {
                          n634 = Decimate 1D Array(w889) -> (w897:u32[], w898:u32[], w895:u32[], w894:u32[], w893:u32[], w892:u32[], w891:u32[], w890:u32[])
                          n635 = for {
                            tunnel: w898 -> [w906] mode=indexing
                            tunnel: w897 -> [w907] mode=indexing
                            tunnel: [w905] -> w896 mode=indexing
                            tunnel: w895 -> [w904] mode=indexing
                            tunnel: w894 -> [w903] mode=indexing
                            tunnel: w893 -> [w902] mode=indexing
                            tunnel: w892 -> [w901] mode=indexing
                            tunnel: w891 -> [w900] mode=indexing
                            tunnel: w890 -> [w899] mode=indexing
                            n636 = Compound Arithmetic op=ADD(w907, w906, w904, w903, w902, w901, w900, w899) -> (w905:u32)
                          }
                        }
                      }
                      n637 = local write "变量：原始数据"(w845) -> ()
                      n638 = local read "变量：感兴区终点道址"() -> (w861:dbl)
                      n639 = local read "变量：感兴区起点道址"() -> (w862:dbl)
                      n640 = for {
                        tunnel: [nan] -> w867 mode=indexing
                        tunnel: w848 -> [_] mode=indexing
                      }
                      n641 = Array Max & Min(array=w848) -> (max value=w852:u32)  [unwired: 3 out]
                      n642 = Multiply(x=w852, y=1.1) -> (x*y=w853:dbl)
                      n643 = Build Array(w848, w867) -> (w863:dbl[][])
                      n644 = local write "变量：图像缓存数组"(w863) -> ()
                      n645 = Index Array(array=w863, index (row)=0 ("索引 (行)")) -> (element=w866:dbl[])  [unwired: 1 in]
                      n646 = Less?(x=w853, y=10.0) -> (x < y?=w854:bool)
                      n647 = case shown="假" w854 {
                        tunnel: w853 -> [w868 _]
                        tunnel: [w868 10.0] -> w849
                        frame False {
                        }
                        frame True {
                        }
                      }
                      n648 = call "一线双色计算.vi"("输入一维数组"=w866, "right corsor"=w861, "left corsor"=w862) -> ("输出波形数组"=w865:dbl[][])
                      n649 = local write "显示：波形图_预览"(w865) -> ()
                      n650 = property on="显示：波形图" class="WFGraph (严格)"("YScale.Maximum"=w849, "YScale.Minimum"=0.0 ("Y标尺.范围:最小值")) -> ()  [unwired: 2 in, 2 out]
                      n651 = property on="显示：波形图_预览" class="WFGraph (严格)"("YScale.Maximum"=w849, "YScale.Minimum"=0.0 ("Y标尺.范围:最小值")) -> ()  [unwired: 2 in, 2 out]
                      n652 = local write "显示：波形图"(w865) -> ()
                    }
                  }
                  n653 = local read "状态：本次测量和上次未完成测量时间和"() -> (w773:dbl)
                  n654 = local read "变量：每次测量计划用时"() -> (w778:u16)
                  n655 = local read "状态：停止变量"() -> (w776:bool)
                  n656 = Greater Or Equal?(x=w773, y=w778) -> (x >= y?=w777:bool)
                  n657 = Or(x=w777, y=w776) -> (x .or. y?=w775:bool)
                }
              }
              frame #2 {
                n658 = flat-sequence {
                  frame #0 {
                    n659 = local write "状态：停止变量"(TRUE ("停止变量")) -> ()
                    n660 = Wait (ms)(milliseconds to wait=u32 100 ("等待时间（毫秒）")) -> ()  [unwired: 1 out]
                  }
                  frame #1 {
                    w943 = T6."Enabled" ("禁用")
                    n661 = local read "变量：上次测量原始数据"() -> (w942:dbl[])
                    n662 = call "MCA_main_read.vi"() -> ("波形图"=w918:i32[])
                    n663 = local read "MCA道宽修正数组"() -> (w925:ext[])
                    n664 = local read "设置：幅度谱总道数"() -> (w941:u32)
                    n665 = local write "状态栏_测量状态"(T3 "停止" ("状态栏_测量状态")) -> ()
                    n666 = local write "状态栏_计数率"(T3 "" ("状态栏_计数率")) -> ()
                    n667 = local write "变量：原始数据"(w918) -> ()
                    n668 = for {
                      tunnel: w918 -> [w1014] mode=indexing
                      tunnel: w942 -> [w1015] mode=indexing
                      tunnel: [w1013] -> w923 mode=indexing
                      n669 = Add(x=w1014, y=w1015) -> (x+y=w1013:dbl)
                    }
                    n670 = Divide(x=8192.0, y=w941) -> (x/y=w939:dbl)
                    n671 = for {
                      tunnel: w925 -> [w971] mode=indexing
                      tunnel: w923 -> [w972] mode=indexing
                      tunnel: [w968] -> w924 mode=indexing
                      n672 = Multiply(x=w972, y=w971) -> (x*y=w970:ext)
                      n673 = Round To Nearest(number=w970) -> (nearest integer value=w969:ext)
                      n674 = To Unsigned Long Integer(number=w969) -> (unsigned 32bit integer=w968:u32)
                    }
                    n675 = local write "变量：上次测量原始数据"(w923) -> ()
                    n676 = case shown="1, 默认" w939 {
                      tunnel: w924 -> [w975 w979 w988 w1003]
                      tunnel: [w975 w976 w985 w1000] -> w932
                      frame 1, Default {
                      }
                      frame 2 {
                        n677 = Decimate 1D Array(w979) -> (w977:u32[], w978:u32[])
                        n678 = for {
                          tunnel: w978 -> [w981] mode=indexing
                          tunnel: w977 -> [w982] mode=indexing
                          tunnel: [w980] -> w976 mode=indexing
                          n679 = Add(x=w982, y=w981) -> (x+y=w980:u32)
                        }
                      }
                      frame 4 {
                        n680 = Decimate 1D Array(w988) -> (w986:u32[], w987:u32[], w984:u32[], w983:u32[])
                        n681 = for {
                          tunnel: w987 -> [w992] mode=indexing
                          tunnel: w986 -> [w993] mode=indexing
                          tunnel: [w991] -> w985 mode=indexing
                          tunnel: w984 -> [w990] mode=indexing
                          tunnel: w983 -> [w989] mode=indexing
                          n682 = Compound Arithmetic op=ADD(w993, w992, w990, w989) -> (w991:u32)
                        }
                      }
                      frame 8 {
                        n683 = Decimate 1D Array(w1003) -> (w1001:u32[], w1002:u32[], w999:u32[], w998:u32[], w997:u32[], w996:u32[], w995:u32[], w994:u32[])
                        n684 = for {
                          tunnel: w1002 -> [w1011] mode=indexing
                          tunnel: w1001 -> [w1012] mode=indexing
                          tunnel: [w1010] -> w1000 mode=indexing
                          tunnel: w999 -> [w1009] mode=indexing
                          tunnel: w998 -> [w1008] mode=indexing
                          tunnel: w997 -> [w1007] mode=indexing
                          tunnel: w996 -> [w1006] mode=indexing
                          tunnel: w995 -> [w1005] mode=indexing
                          tunnel: w994 -> [w1004] mode=indexing
                          n685 = Compound Arithmetic op=ADD(w1012, w1011, w1009, w1008, w1007, w1006, w1005, w1004) -> (w1010:u32)
                        }
                      }
                    }
                    n686 = property on="按钮_开始" class="Bool"("DisabledEnum"=w943) -> ()  [unwired: 2 in, 2 out]
                    n687 = property on="按钮_复位" class="Bool"("DisabledEnum"=w943) -> ()  [unwired: 2 in, 2 out]
                    n688 = property on="按钮_保存" class="Bool"("DisabledEnum"=w943) -> ()  [unwired: 2 in, 2 out]
                    n689 = property on="按钮_设置" class="Bool"("DisabledEnum"=w943) -> ()  [unwired: 2 in, 2 out]
                    n690 = property on="按钮_打开" class="Bool"("DisabledEnum"=w943) -> ()  [unwired: 2 in, 2 out]
                    n691 = property on="按钮_停止" class="Bool (严格)"("DisabledEnum"=T6."Disabled and Grayed Out" ("禁用")) -> ()  [unwired: 2 in, 2 out]
                    n692 = local read "变量：上次测量时间"() -> (w920:dbl)
                    n693 = local read "状态：已测时间"() -> (w921:dbl)
                    n694 = for {
                      tunnel: w932 -> [_] mode=indexing
                      tunnel: [nan] -> w967 mode=indexing
                    }
                    n695 = local read "变量：感兴区起点道址"() -> (w947:dbl)
                    n696 = local read "变量：感兴区终点道址"() -> (w948:dbl)
                    n697 = Array Max & Min(array=w932) -> (max value=w933:u32)  [unwired: 3 out]
                    n698 = Add(x=w921, y=w920) -> (x+y=w919:dbl)
                    n699 = Build Array(w932, w967) -> (w952:dbl[][])
                    n700 = local write "变量：图像缓存数组"(w952) -> ()
                    n701 = local write "变量：上次测量时间"(w919) -> ()
                    n702 = Multiply(x=w933, y=1.1) -> (x*y=w934:dbl)
                    n703 = Index Array(array=w952, index (row)=0 ("索引 (行)")) -> (element=w949:dbl[])  [unwired: 1 in]
                    n704 = Less?(x=w934, y=10.0) -> (x < y?=w935:bool)
                    n705 = call "一线双色计算.vi"("输入一维数组"=w949, "right corsor"=w948, "left corsor"=w947) -> ("输出波形数组"=w950:dbl[][])
                    n706 = case shown="假" w935 {
                      tunnel: w934 -> [w973 _]
                      tunnel: [w973 10.0] -> w929
                      frame False {
                      }
                      frame True {
                      }
                    }
                    n707 = Add Array Elements(numeric array=w932) -> (sum=w938:u32)
                    n708 = Round To Nearest(number=w919) -> (nearest integer value=w922:dbl)
                    n709 = local write "显示：波形图"(w950) -> ()
                    n710 = local write "显示：波形图_预览"(w950) -> ()
                    n711 = Number To Decimal String(number=w919) -> (decimal integer string=w946:string)  [unwired: 1 in]
                    n712 = local read "显示：列表显示内容"() -> (w965:string[])
                    n713 = Divide(x=w938, y=w922) -> (x/y=w954:dbl)
                    n714 = local write "变量 ： 上次测量总计数"(w938) -> ()
                    n715 = Get Date/Time String(date format (0)=enum16{"short", "long", "abbreviated"}."long" ("日期格式(0)"), want seconds? (F)=TRUE ("需要秒？(F)")) -> (date string=w958:string, time string=w957:string)  [unwired: 1 in]
                    n716 = Number To Decimal String(number=w954) -> (decimal integer string=w953:string)  [unwired: 1 in]
                    n717 = Number To Decimal String(number=w938) -> (decimal integer string=w960:string)  [unwired: 1 in]
                    n718 = Concatenate Strings(w946, "秒" ("字符串")) -> (w926:string)
                    n719 = property on="显示：波形图" class="WFGraph (严格)"("YScale.Maximum"=w929, "YScale.Minimum"=0.0 ("Y标尺.范围:最小值")) -> ()  [unwired: 2 in, 2 out]
                    n720 = property on="显示：波形图_预览" class="WFGraph (严格)"("YScale.Maximum"=w929, "YScale.Minimum"=0.0 ("Y标尺.范围:最小值")) -> ()  [unwired: 2 in, 2 out]
                    n721 = Replace Array Subset(array=w965, new element #1=w958, index #1=7 ("索引"), new element #2=w957, index #2=9 ("索引"), new element #3=w960, index #3=10 ("索引"), new element #4=w953, index #4=11 ("索引"), new element #5=w926, index #5=8 ("索引")) -> (w964:string[])
                    n722 = local write "显示：列表显示内容"(w964) -> ()
                  }
                }
              }
              frame #3 {
                n723 = Get Date/Time In Seconds() -> (seconds since 1Jan1904=w1032:timestamp)
                n724 = Get Date/Time String(date format (0)=enum16{"short", "long", "abbreviated"}."long" ("日期格式(0)"), seconds (now)=w1032, want seconds? (F)=TRUE ("需要秒？(F)")) -> (date string=w1033:string, time string=w1022:string)
                n725 = Replace Substring(2:1 ("长度（子字符串长度）"), 3:2 ("偏移量(0)"), 4:"时" ("子字符串(\"\")"), 5:w1022) -> (1:w1020:string)  [unwired: 1 out]
                n726 = Current VI's Path() -> (path=w1045:path)
                n727 = Strip Path(path=w1045) -> (stripped path=w1038:path)  [unwired: 1 out]
                n728 = Replace Substring(2:1 ("长度（子字符串长度）"), 3:6 ("偏移量(0)"), 4:"分" ("子字符串(\"\")"), 5:w1020) -> (1:w1019:string)  [unwired: 1 out]
                n729 = Build Path(base path=w1038, name or relative path="data") -> (appended path=w1036:path)
                n730 = local read "显示：列表显示内容"() -> (w1044:string[])
                n731 = Replace Substring(2:1 ("长度（子字符串长度）"), 3:10 ("偏移量(0)"), 4:"秒" ("子字符串(\"\")"), 5:w1019) -> (1:w1021:string)  [unwired: 1 out]
                n732 = Concatenate Strings(w1033, w1021) -> (w1018:string)
                n733 = Build Path(base path=w1036, name or relative path=w1018) -> (appended path=w1035:path)
                n734 = Index Array(array=w1044, index #1=5 ("索引"), index #2=6 ("索引")) -> (element #1=w1041:string, element #2=w1040:string)
                n735 = property on="列表框" class="MCListbox (严格)"() -> ("ItemNames"=w1058:string[][])  [unwired: 2 in, 2 out]
                n736 = Concatenate Strings(w1041, w1040) -> (w1039:string)
                n737 = TDMS Open(5:FALSE ("创建索引文件？(T)"), 10:T7."create or replace" ("操作(0:open)"), 11:w1035) -> (0:w1050:errorcluster, 3:w1060:refnum<k34>)  [unwired: 4 in]
                n738 = Index Array(array=w1058, index (col)=0 ("禁用的索引 (列)")) -> (element=w1056:string[])  [unwired: 1 in]
                n739 = Replace Array Subset(array=w1044, new element=w1039, index=0 ("索引")) -> (w1055:string[])
                n740 = local write "显示：列表显示内容"(w1055) -> ()
                n741 = Build Array(w1056, w1055) -> (w1047:string[][])
                n742 = TDMS Write(0:w1060, 5:"文件属性" ("组名称输入（无标题）"), 7:string[] ["属性名称", "值"] ("通道名输入（无标题）"), 9:w1047, 11:w1050) -> (4:w1054:refnum<k34>, 15:w1049:errorcluster)  [unwired: 1 in, 2 out]
                n743 = local read "变量：原始数据"() -> (w1046:dbl[])
                n744 = TDMS Write(0:w1054, 5:"数据" ("组名称输入（无标题）"), 7:"计数", 9:w1046, 11:w1049) -> (4:w1051:refnum<k34>, 15:w1048:errorcluster)  [unwired: 1 in, 2 out]
                n745 = TDMS Close(8:w1048, 11:w1051) -> ()  [unwired: 2 out]
              }
            }
          }
        }
      }
    }
  }
  n746 = while {
    stop <- w1066 stop-if-true
    n747 = event shown="[0] 超时" {
      selector: _ -> [_ _]
      dyn-events: _ -> [_ _]
      timeout: 300 -> [_ _]
      tunnel: [_ TRUE] -> w1066
      event Timeout {
        n748 = event-data() -> ()  [unwired: 1 in, 3 out]
        n749 = local read "显示：列表显示内容"() -> (w1075:string[])
        n750 = property on="显示：波形图" class="WFGraph (严格)"("Active Cursor"=u32 0 ("活动游标")) -> (error out=w1073:errorcluster, "Cursor.Visible"=w1072:bool)  [unwired: 2 in, 1 out]
        n751 = property on="列表框" class="MCListbox (严格)"() -> ("ItemNames"=w1087:string[][])  [unwired: 2 in, 2 out]
        n752 = property on="显示：波形图" class="WFGraph (严格)"(error in=w1073) -> (error out=w1070:errorcluster, "Cursor.Cursor X"=w1071:dbl)  [unwired: 1 in, 1 out]
        n753 = Replace Array Subset(array=w1087, new element=w1075, index (col)=1 ("禁用的索引 (列)")) -> (w1088:string[][])  [unwired: 1 in]
        n754 = property on="列表框" class="MCListbox (严格)"("ItemNames"=w1088) -> ()  [unwired: 2 in, 2 out]
        n755 = property on="显示：波形图_预览" class="WFGraph (严格)"(error in=w1070, "Cursor.Cursor X"=w1071) -> ()  [unwired: 1 in, 2 out]
        n756 = case shown="真" w1072 {
          tunnel: w1071 -> [_ w1089]
          tunnel: w1070 -> [_ _]
          frame False {
          }
          frame True {
            n757 = local read "变量：原始数据"() -> (w1092:dbl[])
            n758 = Number To Decimal String(number=w1089) -> (decimal integer string=w1093:string)  [unwired: 1 in]
            n759 = local write "状态栏_游标道址"(w1093) -> ()
            n760 = Index Array(array=w1092, index=w1089) -> (element=w1091:dbl)
            n761 = Number To Decimal String(number=w1091) -> (decimal integer string=w1090:string)  [unwired: 1 in]
            n762 = local write "状态栏_游标计数"(w1090) -> ()
          }
        }
        n763 = UDP Open(11:u16 8080 ("端口")) -> (0:w1068:errorcluster)  [unwired: 4 in, 2 out]
        n764 = Get Date/Time In Seconds() -> (seconds since 1Jan1904=w1085:timestamp)
        n765 = call <vilib>:"Simple Error Handler.vi"("error in (no error)"=w1068) -> ("error?"=w1067:bool)  [unwired: 4 in, 4 out]
        n766 = case shown="假" w1067 {
          tunnel: ["已连接" "未连接"] -> w1076
          frame False {
          }
          frame True {
          }
        }
        n767 = Get Date/Time String(date format (0)=enum16{"short", "long", "abbreviated"}."short" ("日期格式(0)"), seconds (now)=w1085, want seconds? (F)=FALSE ("需要秒？(F)")) -> (date string=w1083:string, time string=w1081:string)
        n768 = Concatenate Strings(w1083, "   " ("字符串"), w1081) -> (→"状态栏_日期":string)
        n769 = Concatenate Strings("核电子学硬件平台" ("字符串"), w1076) -> (→"状态栏_仪器状态":string)
      }
      event "按钮_退出": Value Change; Panel Close {
        n770 = event-data() -> ()  [unwired: 1 in, 3 out]
      }
    }
  }
